vi "Proyecto Final.vi"() -> ()   [LabVIEW 2020]
panel:
  out "km":dbl
  out "ce":dbl
  out "C":dbl
  out "B":dbl
  out "A":dbl
  out "cma":dbl
  out "cpf":dbl
  out "cm":dbl
  out "F gringo":dbl
  out "ks":dbl
  in  "ks como 1":bool
  out "B":dbl
  out "A":dbl
  out "kv":dbl
  out "h gringo":dbl
  out "wt gringa":dbl
  out "v gringa":dbl
  out "dg gringo":dbl
  out "dp gringo":dbl
  out "paso gringo":dbl
  in  "ce engranajes ajusados durante el ensamble":bool
  in  "condicion":u16(ring) items=["Engranajes abiertos", "Unidades comerciales, cerradas", "Unidades de precisión, cerradas", "Unidades de precisión extrema, cerradas"]
  in  "cm op":u16(ring) items=["dientes coronados", "dientes sin coronar"]
  in  "calidad":dbl
  in  "k0":u16(ring) items=["1", "1.25", "1.5", "1.75", "2", "2.25"]
  in  "AGMA":bool
  out "poder h engrane":dbl
  out "Carga wt engrane":dbl
  out "Rall fatiga engrane":dbl
  out "Se g":dbl
  in  "kfg":dbl
  out "kbg":dbl
  out "deg":dbl
  out "tg":dbl
  out "xg":dbl
  out "Con un poder de pipñon h":dbl
  out "Carga que transmite wt piñon":dbl
  out "Rall fatiga piñon":dbl
  out "h otro salon":dbl
  out "wt salon otro":dbl
  out "potencia que puede transmitir diseñado por flexion":dbl
  out "Carga maxima transmitida wt":dbl
  out "radm":dbl
  out "kf":dbl
  out "q final":dbl
  in  "q propuesto":dbl
  out "q calculado":dbl
  in  "que q vas a utilizar":bool
  out "kt final":dbl
  in  "kt propuesto":dbl
  out "kt calculado":dbl
  in  "que kt vas a utilizar":bool
  out "r/d":dbl
  out "rf":dbl
  out "Se":dbl
  out "kb":dbl
  out "de":dbl
  out "t":dbl
  out "ec 14.3":dbl
  out "l":dbl
  out "kaa":dbl
  out "kab":dbl
  out "ka":dbl
  out "H":dbl
  out "rc":dbl
  out "r2":dbl
  out "r1":dbl
  out "Cp":dbl
  in  "Factor de diseño":dbl
  in  "acabado superficial":u16(ring) items=["", "Esmerilado", "Maquinado o laminado en frio", "Laminado en caliente", "Como sale de la forja"]
  out "Seprima":dbl
  out "YG":dbl
  in  "Dureza Brinell":dbl
  in  "Me dan dureza":bool
  in  "Sy":dbl
  in  "Sut":dbl
  in  "me dan el paso?":bool
  out "Caso":i32
  in  "Me dan esfuerzo":bool
  in  "Me dan hp?":bool
  in  "me dan ancho de cara?":bool
  out "Redondeado tabla A-17":dbl
  out "ancho de cara final":dbl
  in  "Tabla 14-8 metrica":dbl[][](array[numeric])=[[0.0, 0.0, 0.0, 0.0, 0.0, 0.0, 0.0], [0.0, 191.0, 181.0, 179.0, 174.0, 162.0, 158.0], [0.0, 181.0, 174.0, 172.0, 168.0, 158.0, 154.0], [0.0, 179.0, 172.0, 170.0, 166.0, 156.0, 152.0], [0.0, 174.0, 168.0, 166.0, 163.0, 154.0, 149.0], [0.0, 162.0, 158.0, 156.0, 154.0, 145.0, 141.0], [0.0, 158.0, 154.0, 152.0, 149.0, 141.0, 137.0]]
  in  "Tabla 14-8 inglesa":dbl[][](array[numeric])=[[0.0, 0.0, 0.0, 0.0, 0.0, 0.0, 0.0], [0.0, 2300.0, 2180.0, 2160.0, 2100.0, 1950.0, 1900.0], [0.0, 2180.0, 2090.0, 2070.0, 2020.0, 1900.0, 1850.0], [0.0, 2160.0, 2070.0, 2050.0, 2000.0, 1880.0, 1830.0], [0.0, 2100.0, 2020.0, 2000.0, 1960.0, 1850.0, 1800.0], [0.0, 1950.0, 1900.0, 1880.0, 1850.0, 1750.0, 1700.0], [0.0, 1900.0, 1850.0, 1830.0, 1800.0, 1700.0, 1650.0]]
  in  "Material de la corona":u16(ring) items=["", "Acero", "Hierro maleable", "Hierro nodular", "Hierro fundido", "Bronce al aluminio", "Bronce al estaño"]
  in  "Material del piñon":u16(ring) items=["", "Acero", "Hierro maleable", "Hierro nodular", "Hierro fundido", "Bronce al aluminio", "Bronce al estaño"]
  out "dG":dbl
  out "paso final":dbl
  out "sigma piñon final":dbl
  out "wt final":dbl
  out "kv final":dbl
  out "Velocidad final":dbl
  out "tabla metrica cuando no te dan ancho de cara 2":string[][](table)=[["0", "0", "0", "0", "0", "0"], ["0", "0", "0", "0", "0", "0"], ["0", "0", "0", "0", "0", "0"], ["0", "0", "000", "0", "0", "0"], ["0", "0", "0", "0", "0", "0"], ["0", "0", "0", "0", "0", "0"], ["0", "0", "00", "0", "0", "0"], ["0", "0", "0", "0", "0", "0"], ["0", "0", "0", "0", "0", "0"], ["0", "0", "0", "0", "0", "0"], ["0", "0", "0", "0", "0", "0"], ["0", "0", "0", "0", "0", "0"], ["0", "0", "0", "0", "0", "0"], ["0", "0", "0", "0", "0", "0"], ["0", "0", "0", "0", "0", "0"], ["0", "0", "0", "0", "0", "0"], ["0", "0", "0", "0", "0", "00"], ["0", "0", "0", "0", "0", "0"], ["0", "0", "0", "0", "0", "0"], ["0", "0", "0", "0", "0", "0"], ["0", "0", "0", "0", "0", "0"], ["0", "0", "0", "0", "0", "0"], ["0", "0", "0", "0", "0", "0"], ["0", "0", "0", "0", "0", "0"], ["0", "0", "0", "0", "0", "0"], ["0", "0", "0", "0", "0", "0"], ["0", "0", "0", "0", "0", "0"], ["0", "0", "0", "0", "0", "0"], ["0", "0", "00", "0", "0", "0"], ["0", "0", "0", "0", "0", "0"], ["0", "0", "0", "0", "0", "0"]]
  in  "Comenzar calculos":bool
  out "Indice tabla":dbl
  in  "Paso predeterminado":dbl
  out "tabla ingles cuando no te dan ancho de cara":string[][](table)=[["0", "0", "0", "0", "0", "0"], ["0", "0", "0", "0", "0", "0"], ["0", "0", "0", "0", "0", "0"], ["0", "0", "000", "0", "0", "0"], ["0", "0", "0", "0", "0", "0"], ["0", "0", "0", "0", "0", "0"], ["0", "0", "00", "0", "0", "0"], ["0", "0", "0", "0", "0", "0"], ["0", "0", "0", "0", "0", "0"], ["0", "0", "0", "0", "0", "0"], ["0", "0", "0", "0", "0", "0"], ["0", "0", "0", "0", "0", "0"], ["0", "0", "0", "0", "0", "0"], ["0", "0", "0", "0", "0", "0"], ["0", "0", "0", "0", "0", "0"], ["0", "0", "0", "0", "0", "0"], ["0", "0", "0", "0", "0", "00"], ["0", "0", "0", "0", "0", "0"], ["0", "0", "0", "0", "0", "0"], ["0", "0", "0", "0", "0", "0"], ["0", "0", "0", "0", "0", "0"], ["0", "0", "0", "0", "0", "0"], ["0", "0", "0", "0", "0", "0"], ["0", "0", "0", "0", "0", "0"], ["0", "0", "0", "0", "0", "0"], ["0", "0", "0", "0", "0", "0"], ["0", "0", "0", "0", "0", "0"], ["0", "0", "0", "0", "0", "0"], ["0", "0", "00", "0", "0", "0"], ["0", "0", "0", "0", "0", "0"], ["0", "0", "0", "0", "0", "0"]]
  out "edfuerxo on":bool
  out "Ancho de cara":dbl
  in  "Esfuerzo permisible":dbl
  in  "stop":bool
  out "Sigma piñon":dbl
  out "Wt":dbl
  out "Kv":dbl
  out "Velocidad":dbl
  out "dp":dbl
  in  "ancho de cara 2":dbl
  in  "hp":dbl
  in  "rpm":dbl
  in  "paso diametral piñon":dbl
  in  "Unidades":T1(radio)
  out "factor de forma de lewizs":string
  out "Y":dbl
  out "resultado dp":string
  out "ancho de cara":string
  in  "dientes corona":dbl
  out "dientes de la corona":string
  out "hp":string
  out "velocidad del piñon":string
  in  "angulo":dbl
  out "angulo":string
  in  "dientes piñon":sgl
  out "dientes del piñon":string
  out "Paso":string
  out "Piñon/corona":string
  # "en watts"
  # "esfuerzo de compresion"
  # "allowable bending stress"
  # "Sensibilidad a la muesca"
  # "esfuerzo admisible"
  # "cosas para sacar kt"
  # "desgaste piñon y engrane"
  # "kc=1"
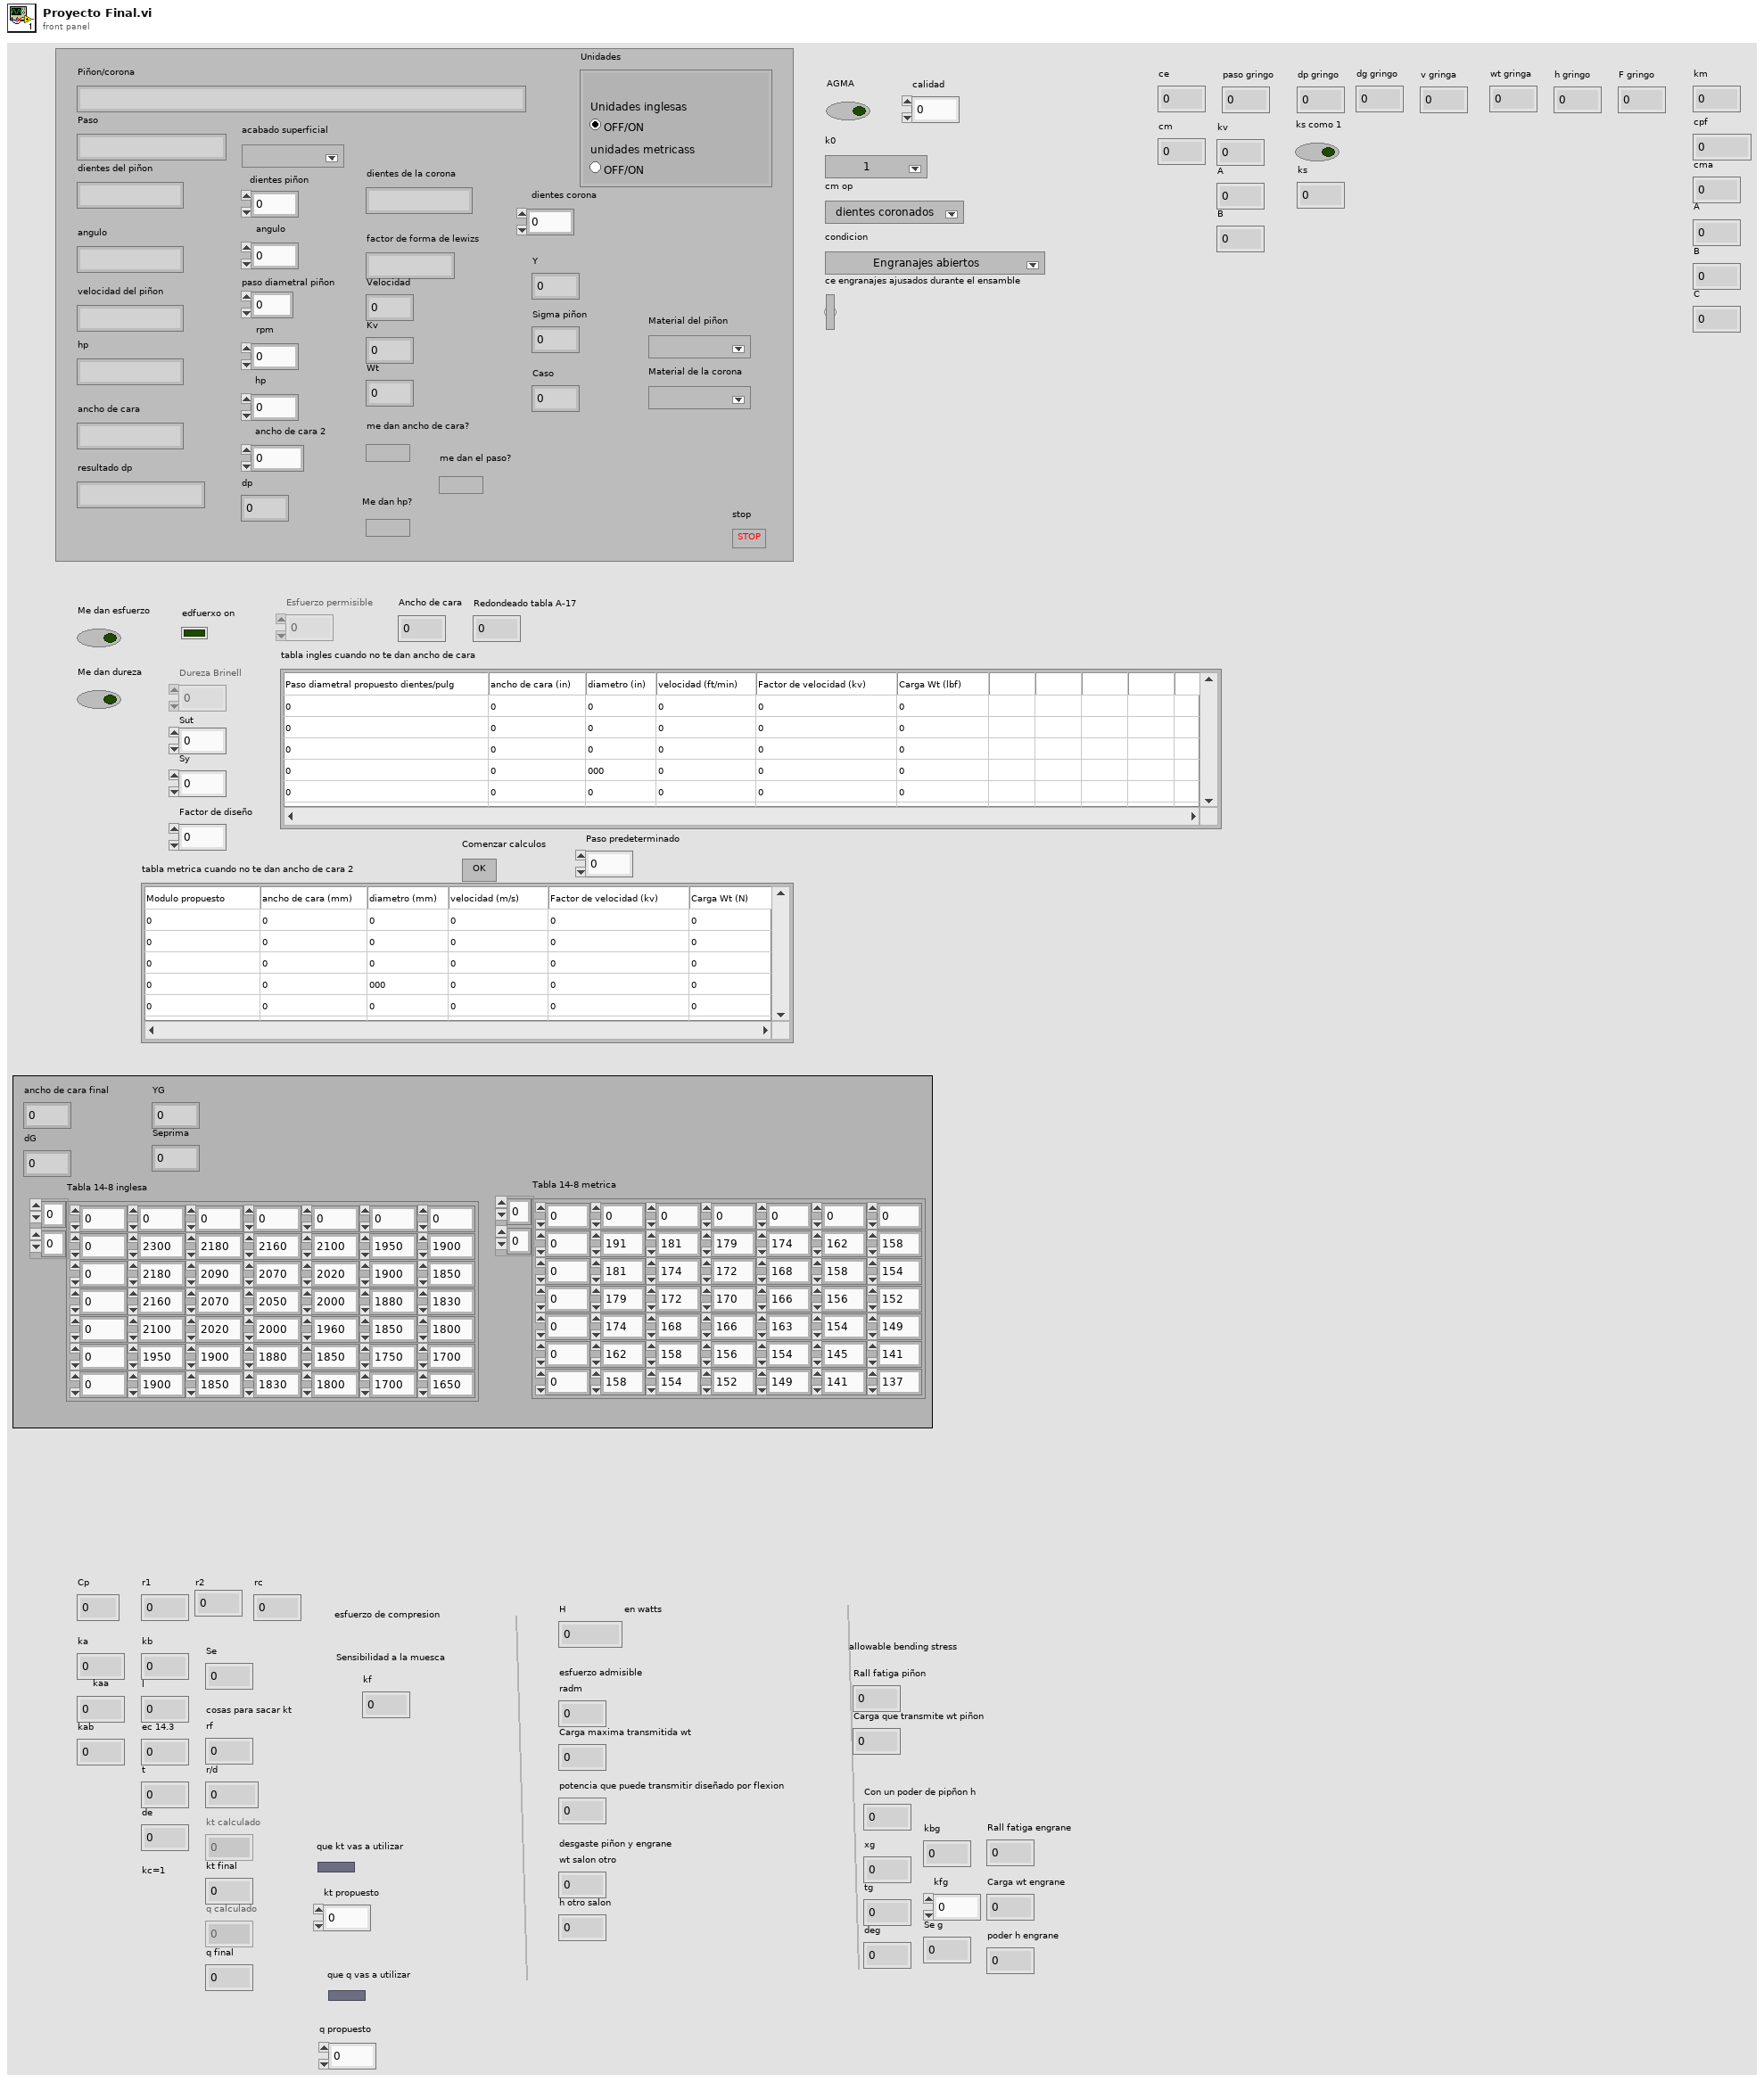
[diagram p1: front panel]
types:
  T1 = enum32{"Unidades inglesas", "unidades metricass"}
  T2 = enum8{"Enabled", "Disabled", "Disabled and Grayed Out"}
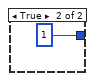
[diagram p2: hidden frame]
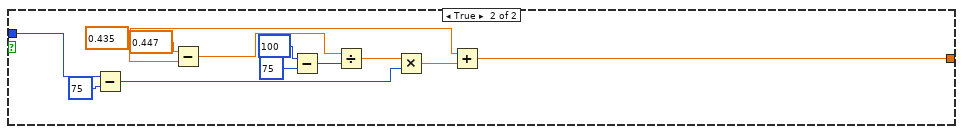
[diagram p3: hidden frame]
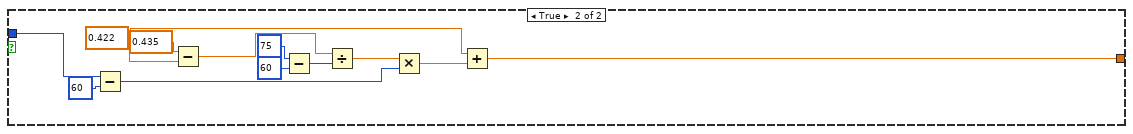
[diagram p4: hidden frame]
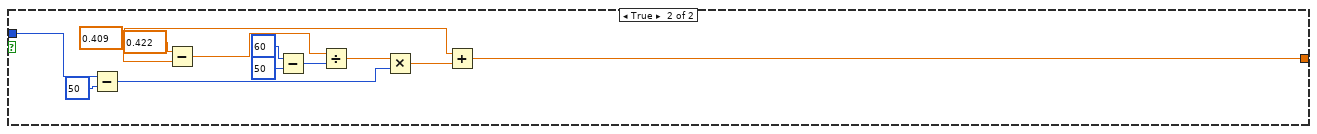
[diagram p5: hidden frame]
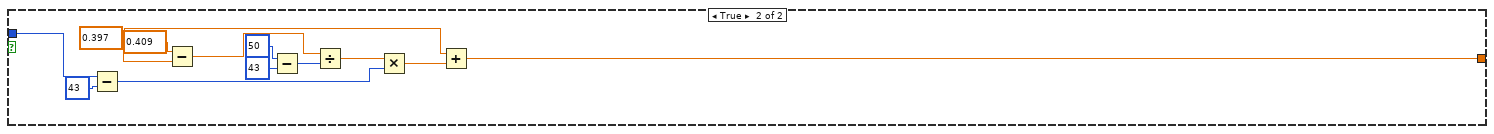
[diagram p6: hidden frame]
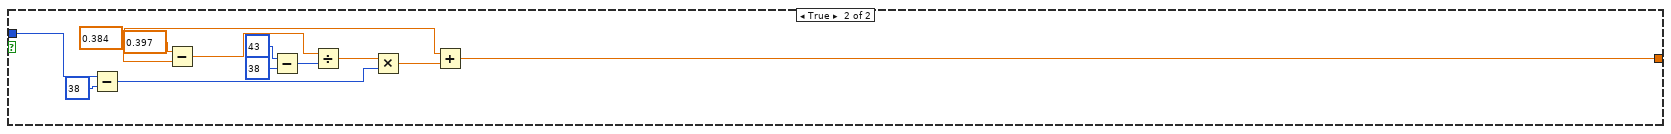
[diagram p7: hidden frame]
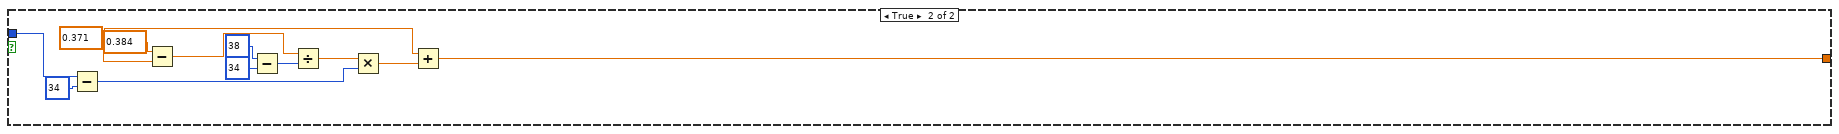
[diagram p8: hidden frame]
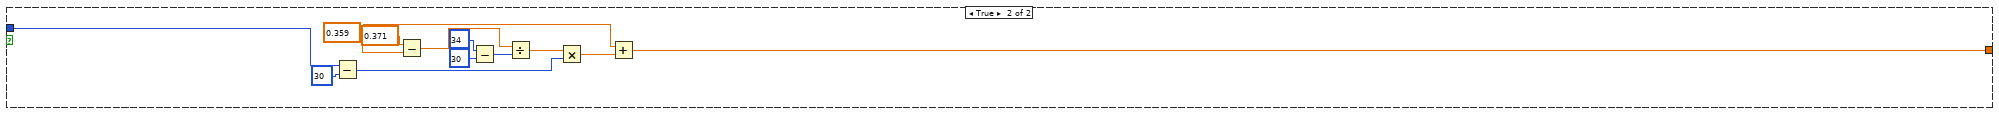
[diagram p9: hidden frame]
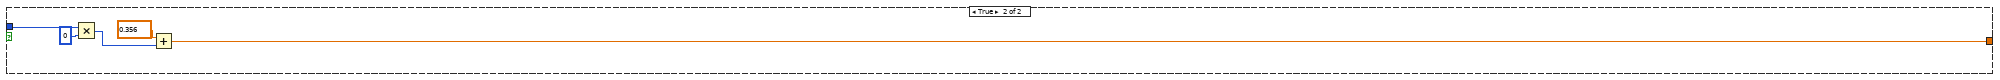
[diagram p10: hidden frame]
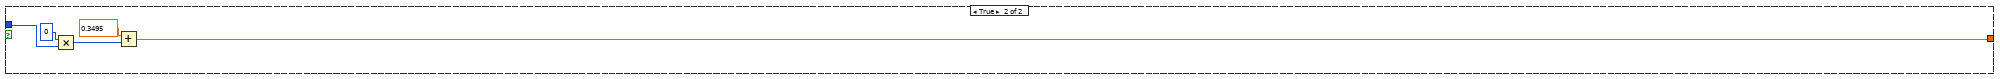
[diagram p11: hidden frame]
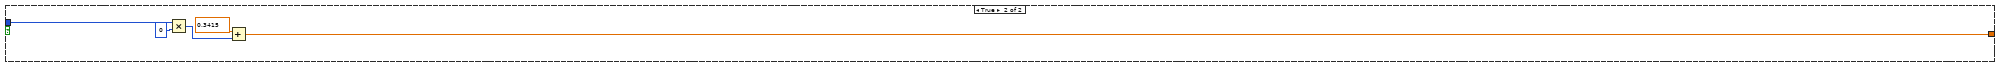
[diagram p12: hidden frame]
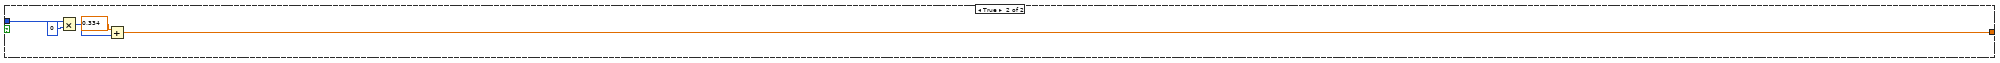
[diagram p13: hidden frame]
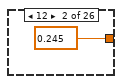
[diagram p14: hidden frame]
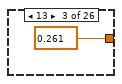
[diagram p15: hidden frame]
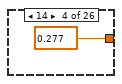
[diagram p16: hidden frame]
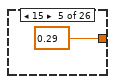
[diagram p17: hidden frame]
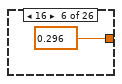
[diagram p18: hidden frame]
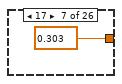
[diagram p19: hidden frame]
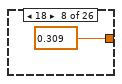
[diagram p20: hidden frame]
diagram:
  n1 = while {
    stop <- "stop" stop-if-true
    # "como lo estoy resolviendo"
    # "Caso: 0 - Me dan todos los datos\nCaso: 1 - No me dan ancho de cara\ncaso 2 - no me dan ni ancho de cara ni paso\ncaso 3 - no me dan hp"
    # "Obtengo Cp y mas cosas"
    # "Me dan todos los datos/no ocupo el sigma extra"
    # "FActor de forma de lewis final"
    # "----------------------------------------------------------------------------------------------------------------------------------------------------------------------------------------------------------------------------------------------------------------------"
    # "Seccion 14-2"
    # "---------------------------------------------------------------------------------------------------------------------------------------------------------------------------------------------------------------------"
    # "DECIDIR CUALES SON LOS DATOS BUENOS"
    # "2 Calculo factor de forma de lewis"
    n2 = local read "Wt"() -> (→"wt final":dbl)
    n3 = local read "Kv"() -> (→"kv final":dbl)
    n4 = local read "Velocidad"() -> (→"Velocidad final":dbl)
    n5 = local read "ancho de cara 2"() -> (→"ancho de cara final":dbl)
    n6 = local read "dientes corona"() -> (w44:dbl)
    n7 = property on="kv final" class="DigNum (strict)"("Visible"=FALSE) -> ()  [unwired: 2 in, 2 out]
    n8 = property on="wt final" class="DigNum (strict)"("Visible"=FALSE) -> ()  [unwired: 2 in, 2 out]
    n9 = property on="paso final" class="DigNum (strict)"("Visible"=FALSE) -> ()  [unwired: 2 in, 2 out]
    n10 = property on="sigma piñon final" class="DigNum (strict)"("Visible"=FALSE) -> ()  [unwired: 2 in, 2 out]
    n11 = property on="Velocidad final" class="DigNum (strict)"("Visible"=FALSE) -> ()  [unwired: 2 in, 2 out]
    n12 = local read "Sigma piñon"() -> (→"sigma piñon final":dbl)
    n13 = local read "paso final"() -> (w43:dbl)
    n14 = local read "Unidades"() -> (w12:T1)
    n15 = local read "angulo"() -> (w40:dbl)
    n16 = local read "dp"() -> (w41:dbl)
    n17 = local read "paso diametral piñon"() -> (→"paso final":dbl)
    n18 = case shown="\"unidades metricass\"" w12 {
      tunnel: w44 -> [w298 w302]
      tunnel: w43 -> [w299 w301]
      tunnel: [w297 w300] -> w13
      frame "Unidades inglesas", Default {
        n19 = formula code="dg=Ng/p;"("p"=w299, "Ng"=w298) -> ("dg"=w297:dbl)
      }
      frame "unidades metricass" {
        # "calcular dg"
        n20 = formula code="dg=Ng*p;"("p"=w301, "Ng"=w302) -> ("dg"=w300:dbl)
      }
    }
    "dG" <- w13
    n21 = local read "dG"() -> (w42:dbl)
    n22 = local read "Caso"() -> (w25:i32)
    n23 = case shown="\"unidades metricass\"" w12 {
      tunnel: "Material de la corona" -> [w974 w985]
      tunnel: "Material del piñon" -> [w975 w984]
      tunnel: [w973 w983] -> w45
      tunnel: w42 -> [w972 w981]
      tunnel: w41 -> [w971 w982]
      tunnel: [w970 w978] -> w46
      tunnel: [w969 w977] -> w47
      tunnel: w40 -> [w967 w980]
      frame "Unidades inglesas", Default {
        n24 = formula code="r1=dp*sin(PHI*(pip/180))/2;\nr2=dg*sin(PHI*(pip/180))/2;"("dg"=w972, "dp"=w971, "PHI"=w967, "pip"=3.141592653589793) -> ("r1"=w970:dbl, "r2"=w969:dbl)
        n25 = Index Array(array="Tabla 14-8 inglesa", index (row)=w975, index (col)=w974) -> (element=w973:dbl)
      }
      frame "unidades metricass" {
        n26 = formula code="r1=dp*sin(PHI*(pip/180))/2;\nr2=dg*sin(PHI*(pip/180))/2;"("dg"=w981, "dp"=w982, "PHI"=w980, "pip"=3.141592653589793) -> ("r1"=w978:dbl, "r2"=w977:dbl)
        n27 = Index Array(array="Tabla 14-8 metrica", index (row)=w984, index (col)=w985) -> (element=w983:dbl)
      }
    }
    "r2" <- w47
    "r1" <- w46
    "Cp" <- w45
    n28 = local read "paso diametral piñon"() -> (w21:dbl)
    n29 = local read "hp"() -> (w22:dbl)
    n30 = local read "Unidades"() -> (w1:T1)
    n31 = case shown="5" w25 {
      tunnel: w1 -> [_ w449 _ _ _ _]
      frame 0, Default {
        # "esfuerzo de compresion"
        n32 = local read "paso diametral piñon"() -> (w367:dbl)
        n33 = local read "ancho de cara 2"() -> (w369:dbl)
        n34 = local read "ancho de cara final"() -> (w362:dbl)
        n35 = local read "Unidades"() -> (w370:T1)
        n36 = local read "kv final"() -> (w359:dbl)
        n37 = local read "Y"() -> (w368:dbl)
        n38 = local read "wt final"() -> (w360:dbl)
        n39 = local read "Wt"() -> (w366:dbl)
        n40 = local read "Kv"() -> (w365:dbl)
        n41 = local read "angulo"() -> (w356:dbl)
        n42 = local read "r1"() -> (w357:dbl)
        n43 = local read "r2"() -> (w358:dbl)
        n44 = local read "Cp"() -> (w355:dbl)
        n45 = case shown="\"unidades metricass\"" w370 {
          tunnel: [w376 w380] -> w364
          tunnel: w365 -> [w375 w388]
          tunnel: w366 -> [w374 w387]
          tunnel: w367 -> [w373 w384]
          tunnel: w369 -> [w372 w385]
          tunnel: w368 -> [w371 w382]
          frame "Unidades inglesas", Default {
            # "paso"
            # "ancho de cara"
            # "sigmapiño"
            # "wt"
            # "kv"
            # "Y"
            # "Paso 6 sacar el esfuerzo de flexion"
            # "Calculo sigma flexion"
            n46 = Multiply(x=w372, y=w371) -> (x*y=w377:dbl)
            n47 = Multiply(x=w375, y=w374) -> (x*y=w379:dbl)
            n48 = Multiply(x=w379, y=w373) -> (x*y=w378:dbl)
            n49 = Divide(x=w378, y=w377) -> (x/y=w376:dbl)
          }
          frame "unidades metricass" {
            # "Y"
            # "paso diametral"
            # "F"
            # "wt"
            # "kv"
            n50 = Multiply(x=w388, y=w387) -> (x*y=w386:dbl)
            n51 = Multiply(x=w384, y=w385) -> (x*y=w383:dbl)
            n52 = Multiply(x=w383, y=w382) -> (x*y=w381:dbl)
            n53 = Divide(x=w386, y=w381) -> (x/y=w380:dbl)
          }
        }
        "Sigma piñon" <- w364
        n54 = formula code="aux2=cos(zy*pip/180);\n//rc=-cp*(((kv*wt)/(f*sin(20*(pip/180)))*(1/r1+1/r2))^(0.5);\nauxiliar1=kv*wt;\nauxiliar2=(1/r1)+(1/r2);\nauxiliar3=((auxiliar1/(aux2*f))*auxiliar2);"("cp"=w355, "kv"=w359, "wt"=w360, "f"=w362, "pip"=3.141592653589793, "r1"=w357, "r2"=w358, "zy"=w356) -> ("auxiliar3"=w353:dbl)  [unwired: 3 out]
        n55 = Negate(x=w355) -> (-x=w361:dbl)
        n56 = Square Root(x=w353) -> (sqrt(x)=w352:dbl)
        n57 = Multiply(x=w361, y=w352) -> (x*y=→"rc":dbl)
      }
      frame 5 {
        n58 = local read "dientes corona"() -> (w445:dbl)
        n59 = local read "dientes piñon"() -> (w447:sgl)
        n60 = local read "paso gringo"() -> (w444:dbl)
        n61 = local read "rpm"() -> (w442:dbl)
        n62 = Subtract(x=12, y="calidad") -> (x-y=w428:dbl)
        n63 = Divide(x=2.0, y=3.0) -> (x/y=w427:dbl)
        n64 = Multiply(x=w442, y=3.141592653589793) -> (x*y=w441:dbl)
        n65 = case shown="True" "ks como 1" {
          tunnel: [w466 1] -> w409
          frame False {
            n66 = local read "Y"() -> (w472:dbl)
            n67 = local read "F gringo"() -> (w473:dbl)
            n68 = Square Root(x=w472) -> (sqrt(x)=w474:dbl)
            n69 = local read "paso gringo"() -> (w470:dbl)
            n70 = Multiply(x=w473, y=w474) -> (x*y=w471:dbl)
            n71 = Divide(x=w471, y=w470) -> (x/y=w469:dbl)
            n72 = Power Of X(1:w469, 2:0.0535 ("y")) -> (0:w468:dbl)
            n73 = Multiply(x=1.192, y=w468) -> (x*y=w466:dbl)
          }
          frame True {
          }
        }
        "ks" <- w409
        n74 = case shown="0, Default" "cm op" {
          tunnel: [0.8 1] -> w392
          frame 0, Default {
          }
          frame 1 {
          }
        }
        "cm" <- w392
        n75 = case shown="False" "ce engranajes ajusados durante el ensamble" {
          tunnel: [1 0.8] -> w398
          frame False {
          }
          frame True {
          }
        }
        "ce" <- w398
        n76 = Power Of X(1:w428, 2:w427) -> (0:w424:dbl)
        n77 = Multiply(x=0.25, y=w424) -> (x*y=w416:dbl)
        "B" <- w416
        n78 = Divide(x=w447, y=w444) -> (x/y=w440:dbl)
        "dp gringo" <- w440
        n79 = Multiply(x=w440, y=w441) -> (x*y=w439:dbl)
        n80 = Divide(x=w439, y=12) -> (x/y=w433:dbl)
        "v gringa" <- w433
        n81 = local read "v gringa"() -> (w412:dbl)
        n82 = Divide(x=w445, y=w444) -> (x/y=→"dg gringo":dbl)
        n83 = Square Root(x=w412) -> (sqrt(x)=w413:dbl)
        n84 = local read "h gringo"() -> (w435:dbl)
        n85 = case shown="\"Unidades inglesas\", Default" w449 {
          tunnel: [w479 w486] -> w448
          tunnel: [w478 w484] -> w436
          tunnel: [w477 w480] -> w408
          frame "Unidades inglesas", Default {
            n86 = local read "paso diametral piñon"() -> (w479:dbl)
            n87 = local read "ancho de cara 2"() -> (w477:dbl)
            n88 = local read "hp"() -> (w478:dbl)
          }
          frame "unidades metricass" {
            # "conviertes todo a inglesas para no batallar"
            n89 = local read "paso diametral piñon"() -> (w488:dbl)
            n90 = local read "hp"() -> (w485:dbl)
            n91 = Multiply(x=25.4, y=w488) -> (x*y=w486:dbl)
            n92 = Multiply(x=w485, y=1.34102) -> (x*y=w484:dbl)
            n93 = local read "ancho de cara 2"() -> (w482:dbl)
            n94 = Divide(x=w482, y=25.4) -> (x/y=w480:dbl)
          }
        }
        "paso gringo" <- w448
        "h gringo" <- w436
        "F gringo" <- w408
        n95 = Subtract(x=1.0, y=w416) -> (x-y=w422:dbl)
        n96 = Multiply(x=w422, y=56) -> (x*y=w420:dbl)
        n97 = local read "A"() -> (w414:dbl)
        n98 = Add(x=w413, y=w414) -> (x+y=w411:dbl)
        n99 = Add(x=w420, y=50) -> (x+y=→"A":dbl)
        n100 = Multiply(x=33000, y=w435) -> (x*y=w434:dbl)
        n101 = Divide(x=w411, y=w414) -> (x/y=w415:dbl)
        n102 = Divide(x=w434, y=w433) -> (x/y=→"wt gringa":dbl)
        n103 = case shown="0, Default" "condicion" {
          tunnel: [0.247 0.127 0.0675 0.0036] -> w405
          tunnel: [0.0167 0.0158 0.0128 0.0102] -> w404
          tunnel: [-7.65e-05 -9.3e-05 -9.26e-05 -8.22e-05] -> w403
          frame 0, Default {
          }
          frame 1 {
          }
          frame 2 {
          }
          frame 3 {
          }
        }
        "A" <- w405
        "B" <- w404
        "C" <- w403
        n104 = local read "dp gringo"() -> (w389:dbl)
        n105 = local read "F gringo"() -> (w402:dbl)
        n106 = Power Of X(1:w415, 2:w416) -> (0:→"kv":dbl)
        n107 = formula code="if(f<=1){\ncpf=(f/(10*d))-0.025;}\nelse{\nif(f<=17){\ncpf=(f/(10*d))-0.0375+(0.0125*f);\n}else{\ncpf=(f/(10*d))-0.1109+(0.0207*f)-(0.000228*f*f);\n}\n}"("f"=w402, "d"=w389) -> ("cpf"=w396:dbl)
        "cpf" <- w396
        n108 = formula code="cma=a+(b*f)+(c*f*f);"("a"=w405, "b"=w404, "c"=w403, "f"=w402) -> ("cma"=w399:dbl)
        "cma" <- w399
        n109 = Multiply(x=w396, y=1) -> (x*y=w394:dbl)
        n110 = Multiply(x=w399, y=w398) -> (x*y=w397:dbl)
        n111 = Add(x=w397, y=w394) -> (x+y=w393:dbl)
        n112 = Multiply(x=w393, y=w392) -> (x*y=w391:dbl)
        n113 = Add(x=1.0, y=w391) -> (x+y=→"km":dbl)
      }
      frame 2 {
        # "si no me dan ancho de cara"
        n114 = case shown="True" "Comenzar calculos" {
          frame False {
          }
          frame True {
            n115 = for {
              N: 30 -> [_]
              i -> [w493]
              # "lo hace invisible"
              n116 = local read "Indice tabla"() -> (w495:dbl)
              n117 = local read "Unidades"() -> (w491:T1)
              n118 = Wait Until Next ms Multiple(millisecond multiple=u32 100) -> ()  [unwired: 1 out]
              n119 = property on="Indice tabla" class="DigNum (strict)"("Visible"=FALSE) -> ()  [unwired: 2 in, 2 out]
              n120 = case shown="\"Unidades inglesas\", Default" w491 {
                tunnel: w495 -> [w496 _]
                frame "Unidades inglesas", Default {
                  # "ancho cara"
                  # "kv"
                  # "carga"
                  # "velocidad"
                  # "paso"
                  # "sistema ingles"
                  n121 = Add(x="Paso predeterminado", y=w496) -> (x+y=w497:dbl)
                  n122 = local read "Esfuerzo permisible"() -> (w501:dbl)
                  n123 = local read "dientes piñon"() -> (w518:sgl)
                  n124 = Multiply(x=w501, y=1000) -> (x*y=w500:dbl)
                  n125 = local read "rpm"() -> (w513:dbl)
                  n126 = local read "hp"() -> (w509:dbl)
                  n127 = local read "Y"() -> (w502:dbl)
                  n128 = formula code="dp=Np/Pd;\nV=(pip*dp*n)/12;\nWt=33000*(H/V);\nkv=(V+1200)/1200;\nF=(kv*Wt*Pd)/(rb*Y);"("Pd"=w497, "Np"=w518, "pip"=3.141592653589793, "n"=w513, "H"=w509, "rb"=w500, "Y"=w502) -> ("dp"=w520:dbl, "V"=w515:dbl, "Wt"=w510:dbl, "kv"=w506:dbl, "F"=w503:dbl)
                  n129 = local read "tabla ingles cuando no te dan ancho de cara"() -> (w525:string[][])
                  n130 = Number To Fractional String(number=w497) -> (F-format string=w523:string)  [unwired: 3 in]
                  n131 = Number To Fractional String(number=w520) -> (F-format string=w519:string)  [unwired: 3 in]
                  n132 = Number To Fractional String(number=w515) -> (F-format string=w516:string)  [unwired: 3 in]
                  n133 = Number To Fractional String(number=w510) -> (F-format string=w511:string)  [unwired: 3 in]
                  n134 = Number To Fractional String(number=w506) -> (F-format string=w507:string)  [unwired: 3 in]
                  n135 = Number To Fractional String(number=w503) -> (F-format string=w504:string)  [unwired: 3 in]
                  n136 = Replace Array Subset "Replace Array Subset"(array=w525, new element #1=w523, index (row) #1=w496, index (col) #1=0 ("disabled index (col)"), new element #2=w519, index (row) #2=w496, index (col) #2=2 ("disabled index (col)"), new element #3=w516, index (row) #3=w496, index (col) #3=3, new element #4=w511, index (row) #4=w496, index (col) #4=5 ("disabled index (col)"), new element #5=w507, index (row) #5=w496, index (col) #5=4 ("disabled index (col)"), new element #6=w504, index (row) #6=w496, index (col) #6=1 ("disabled index (col)")) -> (→"tabla ingles cuando no te dan ancho de cara":string[][])
                }
                frame "unidades metricass" {
                  # "ancho cara"
                  # "kv"
                  # "carga"
                  # "velocidad"
                  # "paso"
                  # "sistema ingles"
                  n137 = local read "Esfuerzo permisible"() -> (w531:dbl)
                  n138 = local read "Paso predeterminado"() -> (w526:dbl)
                  n139 = local read "Indice tabla"() -> (w527:dbl)
                  n140 = local read "dientes piñon"() -> (w528:sgl)
                  n141 = Increment(x=w527) -> (x+1=w552:dbl)
                  n142 = Multiply(x=w531, y=1000) -> (x*y=w534:dbl)
                  n143 = feedback #1(w526) -> (w548:dbl)
                  n144 = feedback-in #1(w552) -> ()
                  n145 = local read "rpm"() -> (w529:dbl)
                  n146 = local read "hp"() -> (w530:dbl)
                  n147 = local read "Y"() -> (w532:dbl)
                  n148 = formula code="dp=Np*Pd;\nV=(pip*dp*n*0.001)/60;\nWt=(H*10000*6)/(dp*0.001*pip*n);\nkv=(V+6.1)/6.1;\nF=(kv*Wt*1000)/(rb*Y*Pd);"("Pd"=w548, "Np"=w528, "pip"=3.141592653589793, "n"=w529, "H"=w530, "rb"=w534, "Y"=w532) -> ("dp"=w550:dbl, "V"=w545:dbl, "Wt"=w541:dbl, "kv"=w538:dbl, "F"=w535:dbl)
                  n149 = local read "tabla metrica cuando no te dan ancho de cara 2"() -> (w556:string[][])
                  n150 = Number To Fractional String(number=w548) -> (F-format string=w554:string)  [unwired: 3 in]
                  n151 = Number To Fractional String(number=w550) -> (F-format string=w549:string)  [unwired: 3 in]
                  n152 = Number To Fractional String(number=w545) -> (F-format string=w546:string)  [unwired: 3 in]
                  n153 = Number To Fractional String(number=w541) -> (F-format string=w542:string)  [unwired: 3 in]
                  n154 = Number To Fractional String(number=w538) -> (F-format string=w539:string)  [unwired: 3 in]
                  n155 = Number To Fractional String(number=w535) -> (F-format string=w536:string)  [unwired: 3 in]
                  n156 = Replace Array Subset "Replace Array Subset"(array=w556, new element #1=w554, index (row) #1=w527, index (col) #1=0 ("disabled index (col)"), new element #2=w549, index (row) #2=w527, index (col) #2=2 ("disabled index (col)"), new element #3=w546, index (row) #3=w527, index (col) #3=3, new element #4=w542, index (row) #4=w527, index (col) #4=5 ("disabled index (col)"), new element #5=w539, index (row) #5=w527, index (col) #5=4 ("disabled index (col)"), new element #6=w536, index (row) #6=w527, index (col) #6=1 ("disabled index (col)")) -> (→"tabla metrica cuando no te dan ancho de cara 2":string[][])
                }
              }
              "Indice tabla" <- w493
            }
          }
        }
      }
      frame 1 {
        n157 = local read "paso diametral piñon"() -> (w562:dbl)
        n158 = local read "Esfuerzo permisible"() -> (w563:dbl)
        n159 = local read "Unidades"() -> (w557:T1)
        n160 = local read "Wt"() -> (w561:dbl)
        n161 = local read "Kv"() -> (w560:dbl)
        n162 = local read "Y"() -> (w564:dbl)
        n163 = case shown="\"Unidades inglesas\", Default" w557 {
          tunnel: w560 -> [w590 w623]
          tunnel: w561 -> [w589 w622]
          tunnel: w563 -> [w587 w620]
          tunnel: w562 -> [w588 w619]
          tunnel: w564 -> [w586 w617]
          tunnel: [w583 w615] -> w559
          frame "Unidades inglesas", Default {
            # "me dieron materiales de los engranes, ergo puedo usar r1"
            n164 = local read "Esfuerzo permisible"() -> (w584:dbl)
            n165 = local read "Cp"() -> (w585:dbl)
            n166 = local read "r2"() -> (w581:dbl)
            n167 = Greater Than 0?(x=w581) -> (x > 0?=w582:bool)
            n168 = case shown="True" w582 {
              tunnel: w590 -> [w601 w612]
              tunnel: w589 -> [w600 w611]
              tunnel: w588 -> [w598 _]
              tunnel: [w597 w602] -> w583
              tunnel: w587 -> [w596 _]
              tunnel: w586 -> [w593 _]
              tunnel: w585 -> [_ w610]
              tunnel: w584 -> [_ w608]
              frame False {
                n169 = Multiply(x=w601, y=w600) -> (x*y=w599:dbl)
                n170 = Multiply(x=1000, y=w596) -> (x*y=w592:dbl)
                n171 = Multiply(x=w599, y=w598) -> (x*y=w594:dbl)
                n172 = Multiply(x=w592, y=w593) -> (x*y=w591:dbl)
                n173 = Divide(x=w594, y=w591) -> (x/y=w597:dbl)
              }
              frame True {
                n174 = Multiply(x=w608, y=1000) -> (x*y=w606:dbl)
                n175 = Divide(x=w610, y=w606) -> (x/y=w609:dbl)
                n176 = local read "angulo"() -> (w605:dbl)
                n177 = Square(x=w609) -> (x^2=w603:dbl)
                n178 = local read "r1"() -> (w614:dbl)
                n179 = local read "r2"() -> (w613:dbl)
                n180 = formula code="invR=(1/r1)+(1/r2);\ninvA=cos(phi*pi/180);\nfrac=(kv*wt)/invA;\nDespejeC=Cuadrado*invR*frac;"("r1"=w614, "r2"=w613, "kv"=w612, "wt"=w611, "phi"=w605, "pi"=3.141592653589793, "Cuadrado"=w603) -> ("DespejeC"=w602:dbl)  [unwired: 3 out]
              }
            }
          }
          frame "unidades metricass" {
            n181 = Multiply(x=w623, y=w622) -> (x*y=w621:dbl)
            n182 = Multiply(x=w619, y=w620) -> (x*y=w618:dbl)
            n183 = Multiply(x=w618, y=w617) -> (x*y=w616:dbl)
            n184 = Divide(x=w621, y=w616) -> (x/y=w615:dbl)
          }
        }
        "Ancho de cara" <- w559
        n185 = case shown="\"unidades metricass\"" w557 {
          tunnel: w559 -> [w566 w577]
          tunnel: [w565 w575] -> w558
          frame "Unidades inglesas", Default {
            n186 = formula code="if(x<=0.01){\n    red=0.01;\n    }else{\n        if(x<=0.012){\n        red=0.012;\n        }else{\n            if(x<=0.016){\n            red=0.016;\n            }else{\n                if(x<=0.02){\n                red=0.02;\n                }else{\n                    if(x<=0.025){\n                    red=0.025;\n                    }else{\n                        if(x<=0.032){\n                        red=0.032;\n                        }else{\n                            if(x<=0.032){\n                            red=0.032;\n                            }else{\n                                if(x<=0.040){\n                                red=0.04;\n                                }else{\n                                    if(x<=0.05){\n                                    red=0.05;\n                                    }else{\n                                        if(x<=0.06){\n                                            red=0.06;\n                                        }else{\n                                            if(x<=0.08){\n                                                red=0.08;\n                                            }else{\n                                               if(x<=0.1){\n                                            red=0.1;\n                                            }else{\n                                        if(x<=0.12){\n                                        red=0.12;\n                                        }else{\n                                    if(x<=0.16){\n                                    red=0.16;\n                                    }else{\n                                if(x<=0.2){\n                                red=0.2;\n                                }else{\n                            if(x<=0.24){\n                            red=0.24;\n                            }else{\n                        if(x<=0.3){\n                        red=0.3;\n                        }else{\n                    if(x<=0.4){\n                    red=0.4;\n                    }else{\n                if(x<=0.5){\n                red=0.5;\n                }else{\n            if(x<=0.6){\n            red=0.6;\n            }else{\n        if(x<=0.8){\n        red=0.8;\n        }else{\n    if(x<=1){\n    red=1;\n    }else{\n    if(x<=1.2){\n        red=1.2;\n    }else{\n        if(x<=1.4){\n            red=1.4;\n        }else{\n            if(x<=1.6){\n                red=1.6;\n            }else{\n                if(x<=1.8){\n                    red=1.8;\n                }else{\n                    if(x<=2){\n                        red=2;\n                    }else{\n                        if(x<=2.6){\n                            red=2.6;\n                        }else{\n                            if(x<=2.8){\n                                red=2.8;\n                            }else{\n                                if(x<=3){\n                                    red=3;\n                                }else{\n                                    if(x<=3.2){\n                                    red=3.2;\n                                    }else{\n                                        if(x<=3.4){\n                                            red=3.4;\n                                        }else{\n                                            if(x<=3.6){\n                                                red=3.6;\n                                            }else{\n                                            if(x<=3.8){\n                                            red=3.8;\n                                            }else{\n                                        if(x<=4){\n                                        red=4;\n                                        }else{\n                                    if(x<=4.2){\n                                    red=4.2;\n                                    }else{\n                                if(x<=4.4){\n                                red=4.4;\n                                }else{\n                            if(x<=4.6){\n                            red=4.6;\n                            }else{\n                                red=x;\n                                        }\n                                    }\n                                }\n                            }\n                        }\n                    }\n                }\n            }\n        }\n    }                                            \n                                            }\n                                        }\n                                    }\n                                }\n                            }\n                        }\n                    }\n                }\n            }\n        }\n    } \n                                            }\n                                        }\n                                    }\n                                }\n                            }\n                        }\n                    }\n                }\n            }\n        }\n    }\n                    }}}}}}"("x"=w566) -> ("red"=w569:dbl)
            n187 = Greater?(x=w569, y=4.6) -> (0:w568:bool)
            n188 = case shown="True" w568 {
              tunnel: [w570 w572] -> w565
              tunnel: w569 -> [w570 w571]
              frame False {
              }
              frame True {
                n189 = formula code="if(x2<=4.8){\n                        red2=4.8;\n                        }else{\n                    if(x2<=5){\n                    red2=5;\n                    }else{\n                if(x2<=5.2){\n                red2=5.2;\n                }else{\n            if(x2<=5.4){\n            red2=5.4;\n            }else{\n        if(x2<=5.6){\n        red2=5.6;\n        }else{\n    if(x2<=5.8){\n    red2=5.8;\n    }else{\nif(x2<=6){\nred2=6;\n}else{\n    if(x2<=7){\n    red2=7;\n    }else{\n        if(x2<=7.5){\n        red2=7.5;\n        }else{\n            if(x2<=8.5){\n            red2=8.5;\n            }else{\n                if(x2<=9){\n                red2=9;\n                }else{\n                    if(x2<=9.5){\n                    red2=9.5;\n                    }else{\n                        if(x2<=10){\n                        red2=10;\n                        }else{\n                            if(x2<=10.5){\n                            red2=10.5;\n                            }else{\n                                if(x2<=11){\n                                red2=11;\n                                }else{\n                                    if(x2<=11.5){\n                                    red2=11.5;\n                                    }else{\n                                        if(x2<=12){\n                                        red2=12;\n                                        }else{\n                                            if(x2<=12.5){\n                                            red2=12.5;\n                                            }else{\n                                        if(x2<=13){\n                                        red2=13;\n                                        }else{\n                                    if(x2<=13.5){\n                                    red2=13.5;\n                                    }else{\n                                if(x2<=14){\n                                red2=14;\n                                }else{\n                            if(x2<=14.5){\n                            red2=14.5;\n                            }else{\n                        if(x2<=15){\n                        red2=15;\n                        }else{\n                    if(x2<=15.5){\n                    red2=15.5;\n                    }else{\n                if(x2<=16){\n                red2=16;\n                }else{\n            if(x2<=16.5){\n            red2=16.5;\n            }else{\n        if(x2<=17){\n        red2=17;\n        }else{\n    if(x2<=17.5){\n    red2=17.5;\n    }else{\nif(x2<=18){\nred2=18;\n}else{\n    if(x2<=18.5){\n    red2=18.5;   \n    }else{\n        if(x2<=19){\n        red2=19;    \n        }else{                                                \n            if(x2<=19.5){\n            red2=19.5;    \n            }else{\n            red2=20;    \n            }\n        }\n                                        }\n                                    }\n                                }\n                            }\n                        }\n                    }\n                }\n            }\n        }\n    }                                            \n                                            }\n                                        }\n                                    }\n                                }\n                            }\n                        }\n                    }\n                }\n            }\n        }\n    } \n                                            }\n                                        }\n                                    }\n                                }\n                            }\n                        }\n                    }\n                }\n            }"("x2"=w571) -> ("red2"=w572:dbl)
              }
            }
          }
          frame "unidades metricass" {
            n190 = formula code="if(x<=0.05){\n    red=0.05;\n    }else{\n        if(x<=0.06){\n        red=0.06;\n        }else{\n            if(x<=0.08){\n            red=0.08;\n            }else{\n                if(x<=0.1){\n                red=0.1;\n                }else{\n                    if(x<=0.12){\n                    red=0.12;\n                    }else{\n                        if(x<=0.16){\n                        red=0.16;\n                        }else{\n                            if(x<=0.2){\n                            red=0.2;\n                            }else{\n                                if(x<=0.25){\n                                red=0.25;\n                                }else{\n                                    if(x<=0.3){\n                                    red=0.3;\n                                    }else{\n                                        if(x<=0.4){\n                                            red=0.4;\n                                        }else{\n                                            if(x<=0.5){\n                                                red=0.5;\n                                            }else{\n                                               if(x<=0.6){\n                                            red=0.6;\n                                            }else{\n                                        if(x<=0.7){\n                                        red=0.7;\n                                        }else{\n                                    if(x<=0.8){\n                                    red=0.8;\n                                    }else{\n                                if(x<=0.9){\n                                red=0.9;\n                                }else{\n                            if(x<=1){\n                            red=1;\n                            }else{\n                        if(x<=1.1){\n                        red=1.1;\n                        }else{\n                    if(x<=1.2){\n                    red=1.2;\n                    }else{\n                if(x<=1.4){\n                red=1.4;\n                }else{\n            if(x<=1.5){\n            red=1.5;\n            }else{\n        if(x<=1.6){\n        red=1.6;\n        }else{\n    if(x<=1.8){\n    red=1.8;\n    }else{\n    if(x<=2){\n        red=2;\n    }else{\n        if(x<=2.2){\n            red=2.2;\n        }else{\n            if(x<=2.5){\n                red=2.5;\n            }else{\n                if(x<=2.8){\n                    red=2.8;\n                }else{\n                    if(x<=3){\n                        red=3;\n                    }else{\n                        if(x<=3.5){\n                            red=3.5;\n                        }else{\n                            if(x<=4){\n                                red=4;\n                            }else{\n                                if(x<=4.5){\n                                    red=4.5;\n                                }else{\n                                    if(x<=5){\n                                    red=5;\n                                    }else{\n                                        if(x<=5.5){\n                                            red=5.5;\n                                        }else{\n                                            if(x<=6){\n                                                red=6;\n                                            }else{\n                                            if(x<=6.5){\n                                            red=6.5;\n                                            }else{\n                                        if(x<=7){\n                                        red=7;\n                                        }else{\n                                    if(x<=8){\n                                    red=8;\n                                    }else{\n                                if(x<=9){\n                                red=9;\n                                }else{\n                            if(x<=10){\n                            red=10;\n                            }else{\n                                red=x;\n                                        }\n                                    }\n                                }\n                            }\n                        }\n                    }\n                }\n            }\n        }\n    }                                            \n                                            }\n                                        }\n                                    }\n                                }\n                            }\n                        }\n                    }\n                }\n            }\n        }\n    } \n                                            }\n                                        }\n                                    }\n                                }\n                            }\n                        }\n                    }\n                }\n            }\n        }\n    }\n                    }}}}}}"("x"=w577) -> ("red"=w576:dbl)
            n191 = Greater?(x=w576, y=10) -> (0:w574:bool)
            n192 = case shown="True" w574 {
              tunnel: [w578 w580] -> w575
              tunnel: w576 -> [w578 w579]
              frame False {
              }
              frame True {
                n193 = formula code="if(x2<=11){\n        red2=11;\n    }else{\n        if(x2<=12){\n        red2=12;\n        }else{\n                if(x2<=14){\n                red2=14;\n                }else{\n                    if(x2<=16){\n                    red2=16;\n                    }else{\n                        if(x2<=18){\n                        red2=18;\n                        }else{\n                            if(x2<=20){\n                            red2=20;\n                            }else{\n                                if(x2<=22){\n                                red2=22;\n                                }else{\n                                    if(x2<=25){\n                                    red2=25;\n                                    }else{\n                                        if(x2<=28){\n                                        red2=28;\n                                        }else{\n                                            if(x2<=30){\n                                            red2=30;    \n                                            }else{\n                                                if(x2<=32){\n                                                red2=32;\n                                                }else{\n                                                    if(x2<=35){\n                                                    red2=35;\n                                                    }else{\n                                                        if(x2<=40){\n                                                        red2=40;\n                                                        }else{\n                                                            if(x2<=45){\n                                                            red2=45;\n                                                            }else{\n                                                                if(x2<=50){\n                                                                red2=50;\n                                                                }else{\n                                                                    if(x2<=60){\n                                                                    red2=60;\n                                                                    }else{\n                                                                        if(x2<=80){\n                                                                        red2=80;\n                                                                        }else{\n                                                                            if(x2<=100){\n                                                                            red2=100;\n                                                                            }else{\n                                                                                if(x2<=120){\n                                                                                red2=120;\n                                                                                }else{\n                                                                                    if(x2<=140){\n                                                                                    red2=140;\n                                                                                    }else{\n                                                                                        if(x2<=160){\n                                                                                        red2=160;\n                                                                                        }else{\n                                                                                            if(x2<=180){\n                                                                                            red2=180;\n                                                                                            }else{\n                                                                                                if(x2<=200){\n                                                                                                red2=200;\n                                                                                                }else{\n                                                                                                    if(x2<=250){\n                                                                                                    red2=250;\n                                                                                                    }else{\n                                                                                                        if(x2<=300){\n                                                                                                        red2=300;\n                                                                                                        }else{\n                                                                                                            red2=x2;\n                                                                                                        }\n                                                                                                    }\n                                                                                                }\n                                                                                            }\n                                                                                        }\n                                                                                    }\n                                                                                }\n                                                                            }\n                                                                        }\n                                                                    }\n                                                                }                                            \n                                                            }\n                                                        }\n                                                    }\n                                                }\n                                            }\n                                        }\n                                    }\n                                }\n                            }\n                        }\n                    } \n                }\n            }\n        }"("x2"=w579) -> ("red2"=w580:dbl)
              }
            }
          }
        }
        "Redondeado tabla A-17" <- w558
      }
      frame 3 {
        w631 = 3.141592653589793
        # "wt"
        n194 = local read "ancho de cara 2"() -> (w625:dbl)
        n195 = local read "Unidades"() -> (w627:T1)
        n196 = local read "Esfuerzo permisible"() -> (w626:dbl)
        n197 = local read "Cp"() -> (w640:dbl)
        n198 = local read "angulo"() -> (w637:dbl)
        n199 = local read "r2"() -> (w639:dbl)
        n200 = local read "Kv"() -> (w636:dbl)
        n201 = local read "r1"() -> (w638:dbl)
        n202 = case shown="\"unidades metricass\"" w627 {
          tunnel: w625 -> [w641 w644]
          tunnel: [w641 w643] -> w624
          frame "Unidades inglesas", Default {
          }
          frame "unidades metricass" {
            n203 = Multiply(x=0.001, y=w644) -> (x*y=w643:dbl)
          }
        }
        n204 = formula code="cedos=RC/CP;\nREINV=(1/R1)+(1/R2);\npor=F*cos(PHI*pi/180);\nWet=por/(REINV*kev);"("RC"=w626, "CP"=w640, "F"=w624, "PHI"=w637, "R1"=w638, "R2"=w639, "pi"=w631, "kev"=w636) -> ("Wet"=w634:dbl, "cedos"=w635:dbl)  [unwired: 2 out]
        n205 = Square(x=w635) -> (x^2=w633:dbl)
        n206 = Multiply(x=w633, y=w634) -> (x*y=w632:dbl)
        n207 = local read "dp"() -> (w630:dbl)
        n208 = local read "rpm"() -> (w628:dbl)
        n209 = formula code="H=(wet*pi*dep*nep)/60;"("wet"=w632, "pi"=w631, "dep"=w630, "nep"=w628) -> ("H"=→"H":dbl)
      }
      frame 4 {
        # "cosas que pide el problema 14-18 --------------------------------------------------------------------------------------------------------------------------------------------------"
        # "esfuerzo permisible"
        # "ecuacion 6-32"
        # "kf = 1.66"
        # "Determinar kb"
        # "DEterminar Ka"
        n210 = local read "Factor de diseño"() -> (w653:dbl)
        n211 = local read "paso diametral piñon"() -> (w732:dbl)
        n212 = Greater Than 0?(x="Sut") -> (x > 0?=w685:bool)
        n213 = case shown="False" w685 {
          tunnel: [w751 w754] -> w684
          tunnel: "Sut" -> [_ w754]
          frame False {
            n214 = local read "Dureza Brinell"() -> (w752:dbl)
            n215 = Multiply(x=0.5, y=w752) -> (x*y=w751:dbl)
          }
          frame True {
          }
        }
        n216 = local read "Se"() -> (w678:dbl)
        n217 = local read "Seprima"() -> (w727:dbl)
        n218 = local read "kb"() -> (w726:dbl)
        n219 = local read "ka"() -> (w728:dbl)
        n220 = Multiply(x=w684, y=0.5) -> (x*y=→"Seprima":dbl)
        n221 = Multiply(x=w727, y=w728) -> (x*y=w725:dbl)
        n222 = Divide(x=w678, y=w653) -> (x/y=w677:dbl)
        "Rall fatiga piñon" <- w677
        n223 = Multiply(x=w725, y=w726) -> (x*y=w723:dbl)
        n224 = local read "paso diametral piñon"() -> (w648:dbl)
        n225 = local read "ancho de cara 2"() -> (w651:dbl)
        n226 = Multiply(x=w723, y=1.66) -> (x*y=→"Se":dbl)
        n227 = local read "Unidades"() -> (w691:T1)
        n228 = local read "Velocidad"() -> (w647:dbl)
        n229 = local read "Kv"() -> (w649:dbl)
        n230 = local read "Y"() -> (w679:dbl)
        n231 = case shown="\"Unidades inglesas\", Default" w691 {
          tunnel: [w896 w921] -> w733
          tunnel: w732 -> [w900 w927]
          tunnel: [w894 w920] -> w731
          tunnel: [w892 w918] -> w718
          tunnel: [w885 w911] -> w730
          tunnel: [w884 w913] -> w729
          frame "Unidades inglesas", Default {
            n232 = formula code="L=(1/pd)+(1.25/pd);"("pd"=w900) -> ("L"=w896:dbl)
            n233 = local read "paso diametral piñon"() -> (w898:dbl)
            n234 = local read "Y"() -> (w899:dbl)
            n235 = formula code="equis=(3*yp)/(2*pe);"("yp"=w899, "pe"=w898) -> ("equis"=w894:dbl)
            n236 = Multiply(x=4, y=w896) -> (x*y=w895:dbl)
            n237 = Multiply(x=w895, y=w894) -> (x*y=w893:dbl)
            n238 = local read "ancho de cara 2"() -> (w891:dbl)
            n239 = Square Root(x=w893) -> (sqrt(x)=w892:dbl)
            n240 = Multiply(x=w891, y=w892) -> (x*y=w890:dbl)
            n241 = Square Root(x=w890) -> (sqrt(x)=w889:dbl)
            n242 = Multiply(x=0.808, y=w889) -> (x*y=w885:dbl)
            n243 = Less Or Equal?(x=w885, y=2.0) -> (x <= y?=w887:bool)
            n244 = case shown="True" w887 {
              tunnel: w885 -> [w902 w910]
              tunnel: [w901 w906] -> w884
              frame False {
                n245 = Power Of X(1:w902, 2:-0.157 ("y")) -> (0:w904:dbl)
                n246 = Multiply(x=w904, y=0.91) -> (x*y=w901:dbl)
              }
              frame True {
                n247 = Power Of X(1:w910, 2:-0.107 ("y")) -> (0:w908:dbl)
                n248 = Multiply(x=w908, y=0.879) -> (x*y=w906:dbl)
              }
            }
          }
          frame "unidades metricass" {
            n249 = local read "paso diametral piñon"() -> (w925:dbl)
            n250 = formula code="L=(1*pd)+(1.25*pd);"("pd"=w927) -> ("L"=w921:dbl)
            n251 = local read "Y"() -> (w926:dbl)
            n252 = formula code="equis=(3*yp*pe)/2;"("yp"=w926, "pe"=w925) -> ("equis"=w920:dbl)
            n253 = Multiply(x=4, y=w921) -> (x*y=w924:dbl)
            n254 = Multiply(x=w924, y=w920) -> (x*y=w923:dbl)
            n255 = Square Root(x=w923) -> (sqrt(x)=w918:dbl)
            n256 = local read "ancho de cara 2"() -> (w919:dbl)
            n257 = Multiply(x=w919, y=w918) -> (x*y=w917:dbl)
            n258 = Square Root(x=w917) -> (sqrt(x)=w916:dbl)
            n259 = Multiply(x=0.808, y=w916) -> (x*y=w911:dbl)
            n260 = Less Or Equal?(x=w911, y=51) -> (x <= y?=w914:bool)
            n261 = case shown="False" w914 {
              tunnel: w911 -> [w929 w936]
              tunnel: [w928 w933] -> w913
              frame False {
                n262 = Power Of X(1:w929, 2:-0.157) -> (0:w930:dbl)
                n263 = Multiply(x=1.51, y=w930) -> (x*y=w928:dbl)
              }
              frame True {
                n264 = Power Of X(1:w936, 2:-0.107) -> (0:w934:dbl)
                n265 = Multiply(x=1.24, y=w934) -> (x*y=w933:dbl)
              }
            }
          }
        }
        "l" <- w733
        "ec 14.3" <- w731
        "t" <- w718
        "de" <- w730
        "kb" <- w729
        n266 = local read "paso diametral piñon"() -> (w720:dbl)
        n267 = local read "YG"() -> (w650:dbl)
        n268 = case shown="2" "acabado superficial" {
          tunnel: w691 -> [_ w941 w944 w949 w954]
          tunnel: [w938 w940 w946 w951 w956] -> w735
          tunnel: [w938 -0.265 -0.718 -0.995 -0.085] -> w738
          frame 0, Default {
            w938 = 0
          }
          frame 2 {
            n269 = case shown="\"Unidades inglesas\", Default" w941 {
              tunnel: [2.7 4.51] -> w940
              frame "Unidades inglesas", Default {
              }
              frame "unidades metricass" {
              }
            }
          }
          frame 3 {
            n270 = case shown="\"unidades metricass\"" w944 {
              tunnel: [14.4 57.7] -> w946
              frame "Unidades inglesas", Default {
              }
              frame "unidades metricass" {
              }
            }
          }
          frame 4 {
            n271 = case shown="\"unidades metricass\"" w949 {
              tunnel: [39.9 272] -> w951
              frame "Unidades inglesas", Default {
              }
              frame "unidades metricass" {
              }
            }
          }
          frame 1 {
            n272 = case shown="\"unidades metricass\"" w954 {
              tunnel: [1.34 1.58] -> w956
              frame "Unidades inglesas", Default {
              }
              frame "unidades metricass" {
              }
            }
          }
        }
        "kab" <- w738
        "kaa" <- w735
        n273 = formula code="wt=(F*y*rall)/(kv*pd);\nhp=(wt*v)/33;"("F"=w651, "y"=w679, "rall"=w677, "kv"=w649, "pd"=w648, "v"=w647) -> ("wt"=→"Carga que transmite wt piñon":dbl, "hp"=→"Con un poder de pipñon h":dbl)
        n274 = case shown="False" "que kt vas a utilizar" {
          tunnel: [T2."Disabled and Grayed Out" ("Disabled") T2."Enabled" ("Disabled")] -> w715
          tunnel: [T2."Enabled" ("Disabled") T2."Disabled and Grayed Out" ("Disabled")] -> w714
          tunnel: [w874 "kt propuesto"] -> w710
          frame False {
            n275 = local read "r/d"() -> (w878:dbl)
            n276 = Power Of X(1:w878, 2:-0.33333) -> (0:w876:dbl)
            n277 = Multiply(x=0.9072, y=w876) -> (x*y=w874:dbl)
            "kt calculado" <- w874
          }
          frame True {
          }
        }
        "kt final" <- w710
        n278 = case shown="\"unidades metricass\"" w691 {
          tunnel: 0.3 -> [w845 w849]
          tunnel: w720 -> [w844 w848]
          tunnel: [w846 w847] -> w719
          frame "Unidades inglesas", Default {
            n279 = Divide(x=w845, y=w844) -> (x/y=w846:dbl)
          }
          frame "unidades metricass" {
            n280 = Multiply(x=w849, y=w848) -> (x*y=w847:dbl)
          }
        }
        "rf" <- w719
        n281 = Power Of X(1:w684, 2:w738) -> (0:w736:dbl)
        n282 = Divide(x=w719, y=w718) -> (x/y=→"r/d":dbl)
        n283 = local read "Sut"() -> (w688:dbl)
        n284 = Multiply(x=w736, y=w735) -> (x*y=→"ka":dbl)
        n285 = Greater Than 0?(x=w688) -> (x > 0?=w689:bool)
        n286 = property on="kt calculado" class="DigNum (strict)"("DisabledEnum"=w714) -> ()  [unwired: 2 in, 2 out]
        n287 = property on="kt propuesto" class="DigNum (strict)"("DisabledEnum"=w715) -> ()  [unwired: 2 in, 2 out]
        n288 = case shown="True" w689 {
          tunnel: [w755 w760] -> w687
          tunnel: "Factor de diseño" -> [w756 w758]
          frame False {
            n289 = Divide(x="Sy", y=w756) -> (x/y=w755:dbl)
          }
          frame True {
            n290 = local read "Se"() -> (w762:dbl)
            n291 = local read "kf"() -> (w761:dbl)
            n292 = Multiply(x=w761, y=w758) -> (x*y=w759:dbl)
            n293 = Divide(x=w762, y=w759) -> (x/y=w760:dbl)
          }
        }
        "radm" <- w687
        n294 = case shown="False" "que q vas a utilizar" {
          tunnel: [T2."Disabled and Grayed Out" ("Disabled") T2."Enabled" ("Disabled")] -> w712
          tunnel: [T2."Enabled" ("Disabled") T2."Disabled and Grayed Out" ("Disabled")] -> w711
          tunnel: [w855 "q propuesto"] -> w709
          frame False {
            n295 = local read "Unidades"() -> (w854:T1)
            n296 = local read "Sut"() -> (w852:dbl)
            n297 = local read "rf"() -> (w851:dbl)
            n298 = case shown="\"unidades metricass\"" w854 {
              tunnel: [w864 w868] -> w853
              tunnel: w852 -> [w864 w870]
              tunnel: w851 -> [w863 w867]
              tunnel: [w863 w865] -> w850
              frame "Unidades inglesas", Default {
              }
              frame "unidades metricass" {
                n299 = Divide(x=w870, y=6.895) -> (x/y=w868:dbl)
                n300 = Divide(x=w867, y=25.4) -> (x/y=w865:dbl)
              }
            }
            n301 = Square Root(x=w850) -> (sqrt(x)=w857:dbl)
            n302 = Square(x=w853) -> (x^2=w860:dbl)
            n303 = Power Of X(1:w853, 2:3) -> (0:w859:dbl)
            n304 = formula code="Ra=0.246-(0.00308*sut1)+(0.0000151*sut2)-(0.0000000267*sut3);"("sut1"=w853, "sut2"=w860, "sut3"=w859) -> ("Ra"=w856:dbl)
            n305 = formula code="q=1/(1+(Ra/Rr));"("Rr"=w857, "Ra"=w856) -> ("q"=w855:dbl)
            "q calculado" <- w855
          }
          frame True {
          }
        }
        "q final" <- w709
        n306 = local read "paso diametral piñon"() -> (w674:dbl)
        n307 = formula code="kf=1+(q*(kt-1));"("kt"=w710, "q"=w709) -> ("kf"=→"kf":dbl)
        n308 = local read "YG"() -> (w675:dbl)
        n309 = local read "ancho de cara 2"() -> (w698:dbl)
        n310 = formula code="equis=(3*yg)/(2*pe);"("yg"=w675, "pe"=w674) -> ("equis"=w670:dbl)
        "xg" <- w670
        n311 = local read "paso diametral piñon"() -> (w696:dbl)
        n312 = local read "Y"() -> (w697:dbl)
        n313 = local read "l"() -> (w669:dbl)
        n314 = local read "Kv"() -> (w695:dbl)
        n315 = local read "Velocidad"() -> (w692:dbl)
        n316 = Multiply(x=4, y=w669) -> (x*y=w672:dbl)
        n317 = Multiply(x=w672, y=w670) -> (x*y=w671:dbl)
        n318 = local read "ancho de cara 2"() -> (w664:dbl)
        n319 = Square Root(x=w671) -> (sqrt(x)=w665:dbl)
        "tg" <- w665
        n320 = case shown="\"Unidades inglesas\", Default" w691 {
          tunnel: w698 -> [w818 w842]
          tunnel: w687 -> [w819 w837]
          tunnel: w697 -> [w817 w841]
          tunnel: w696 -> [w815 w839]
          tunnel: w695 -> [w816 w835]
          tunnel: [w812 w834] -> w694
          tunnel: [w813 w831] -> w693
          tunnel: w692 -> [w814 _]
          frame "Unidades inglesas", Default {
            n321 = Multiply(x=w819, y=w818) -> (x*y=w826:dbl)
            n322 = Multiply(x=w826, y=w817) -> (x*y=w824:dbl)
            n323 = Multiply(x=w816, y=w815) -> (x*y=w825:dbl)
            n324 = Divide(x=w824, y=w825) -> (x/y=w812:dbl)
            n325 = Multiply(x=1000, y=w812) -> (x*y=w823:dbl)
            n326 = Multiply(x=w823, y=w814) -> (x*y=w822:dbl)
            n327 = Divide(x=w822, y=33000) -> (x/y=w813:dbl)
          }
          frame "unidades metricass" {
            # "dp/2"
            n328 = local read "rpm"() -> (w830:dbl)
            n329 = local read "dp"() -> (w829:dbl)
            n330 = Multiply(x=w842, y=w841) -> (x*y=w840:dbl)
            n331 = Multiply(x=w840, y=w839) -> (x*y=w838:dbl)
            n332 = Divide(x=w829, y=2) -> (x/y=w827:dbl)
            n333 = Multiply(x=w838, y=w837) -> (x*y=w836:dbl)
            n334 = Divide(x=w836, y=w835) -> (x/y=w834:dbl)
            n335 = Multiply(x=w834, y=w830) -> (x*y=w833:dbl)
            n336 = Multiply(x=w833, y=w827) -> (x*y=w832:dbl)
            n337 = Divide(x=w832, y=9550000) -> (x/y=w831:dbl)
          }
        }
        "Carga maxima transmitida wt" <- w694
        "potencia que puede transmitir diseñado por flexion" <- w693
        n338 = Multiply(x=w664, y=w665) -> (x*y=w668:dbl)
        n339 = Square Root(x=w668) -> (sqrt(x)=w667:dbl)
        n340 = Multiply(x=0.808, y=w667) -> (x*y=w661:dbl)
        "deg" <- w661
        n341 = Less Or Equal?(x=w661, y=2.0) -> (x <= y?=w662:bool)
        n342 = local read "ancho de cara 2"() -> (w704:dbl)
        n343 = property on="q calculado" class="DigNum (strict)"("DisabledEnum"=w711) -> ()  [unwired: 2 in, 2 out]
        n344 = property on="q propuesto" class="DigNum (strict)"("DisabledEnum"=w712) -> ()  [unwired: 2 in, 2 out]
        n345 = case shown="True" w662 {
          tunnel: w661 -> [w742 w750]
          tunnel: [w741 w746] -> w660
          frame False {
            n346 = Power Of X(1:w742, 2:-0.157 ("y")) -> (0:w744:dbl)
            n347 = Multiply(x=w744, y=0.91) -> (x*y=w741:dbl)
          }
          frame True {
            n348 = Power Of X(1:w750, 2:-0.107 ("y")) -> (0:w748:dbl)
            n349 = Multiply(x=w748, y=0.879) -> (x*y=w746:dbl)
          }
        }
        "kbg" <- w660
        n350 = local read "angulo"() -> (w681:dbl)
        n351 = local read "r1"() -> (w702:dbl)
        n352 = local read "r2"() -> (w703:dbl)
        n353 = local read "Kv"() -> (w680:dbl)
        n354 = local read "Cp"() -> (w707:dbl)
        n355 = local read "Factor de diseño"() -> (w705:dbl)
        n356 = Multiply(x=w660, y="kfg") -> (x*y=w658:dbl)
        n357 = local read "Seprima"() -> (w655:dbl)
        n358 = local read "ka"() -> (w657:dbl)
        n359 = Multiply(x=w658, y=w657) -> (x*y=w656:dbl)
        n360 = Multiply(x=w656, y=w655) -> (x*y=w654:dbl)
        "Se g" <- w654
        n361 = Divide(x=w654, y=w653) -> (x/y=w652:dbl)
        "Rall fatiga engrane" <- w652
        n362 = formula code="wtg=(F*y*rall)/(kv*pd);\nhpg=(wtg*v)/33;"("F"=w651, "y"=w650, "rall"=w652, "kv"=w649, "pd"=w648, "v"=w647) -> ("wtg"=→"Carga wt engrane":dbl, "hpg"=→"poder h engrane":dbl)
        n363 = local read "Velocidad"() -> (w690:dbl)
        n364 = case shown="\"Unidades inglesas\", Default" w691 {
          tunnel: w707 -> [w772 w811]
          tunnel: "Dureza Brinell" -> [w774 w810]
          tunnel: w705 -> [w773 w804]
          tunnel: w704 -> [w771 w800]
          tunnel: w681 -> [w770 w799]
          tunnel: w703 -> [w768 w798]
          tunnel: w702 -> [w769 w797]
          tunnel: w680 -> [w767 w796]
          tunnel: 3.141592653589793 -> [w766 w795]
          tunnel: [w765 w791] -> w700
          tunnel: [w763 w789] -> w699
          tunnel: w690 -> [w764 _]
          frame "Unidades inglesas", Default {
            n365 = Multiply(x=0.4, y=w774) -> (x*y=w784:dbl)
            n366 = Subtract(x=w784, y=10) -> (x-y=w782:dbl)
            n367 = Multiply(x=w782, y=1000) -> (x*y=w780:dbl)
            n368 = Square Root(x=w773) -> (sqrt(x)=w779:dbl)
            n369 = Divide(x=w780, y=w779) -> (x/y=w778:dbl)
            n370 = formula code="cedos=RC/CP;\nREINV=(1/R1)+(1/R2);\npor=F*cos(PHI*pi/180);\nWet=por/(REINV*kev);"("RC"=w778, "CP"=w772, "F"=w771, "PHI"=w770, "R1"=w769, "R2"=w768, "pi"=w766, "kev"=w767) -> ("Wet"=w776:dbl, "cedos"=w777:dbl)  [unwired: 2 out]
            n371 = Square(x=w777) -> (x^2=w775:dbl)
            n372 = Multiply(x=w775, y=w776) -> (x*y=w765:dbl)
            n373 = formula code="H=(wet*V)/33000;"("wet"=w765, "V"=w764) -> ("H"=w763:dbl)
          }
          frame "unidades metricass" {
            n374 = Multiply(x=0.4, y=w810) -> (x*y=w808:dbl)
            n375 = Subtract(x=w808, y=10) -> (x-y=w806:dbl)
            n376 = Multiply(x=w806, y=6.89) -> (x*y=w803:dbl)
            n377 = Square Root(x=w804) -> (sqrt(x)=w802:dbl)
            n378 = Divide(x=w803, y=w802) -> (x/y=w801:dbl)
            n379 = formula code="cedos=RC/CP;\nREINV=(1/R1)+(1/R2);\npor=F*cos(PHI*pi/180);\nWet=por/(REINV*kev);"("RC"=w801, "CP"=w811, "F"=w800, "PHI"=w799, "R1"=w797, "R2"=w798, "pi"=w795, "kev"=w796) -> ("Wet"=w793:dbl, "cedos"=w794:dbl)  [unwired: 2 out]
            n380 = Square(x=w794) -> (x^2=w792:dbl)
            n381 = Multiply(x=w792, y=w793) -> (x*y=w791:dbl)
            n382 = local read "dp"() -> (w790:dbl)
            n383 = local read "rpm"() -> (w787:dbl)
            n384 = formula code="T=(wet*V)/2;\nH=(T*fast)/9.55;"("wet"=w791, "V"=w790, "fast"=w787) -> ("H"=w786:dbl)  [unwired: 1 out]
            n385 = Divide(x=w786, y=1000000.0) -> (x/y=w789:dbl)
          }
        }
        "wt salon otro" <- w700
        "h otro salon" <- w699
      }
    }
    n386 = local read "rpm"() -> (w20:dbl)
    n387 = case shown="\"unidades metricass\"" w1 {
      tunnel: ["paso diametral" "módulo"] -> w24
      tunnel: ["Fuerza que transmite" "Carga fija que soporta"] -> w23
      tunnel: w21 -> [w303 w344]
      tunnel: [w312 w323] -> w17
      tunnel: w20 -> [w311 w331]
      tunnel: [w306 w327] -> w18
      tunnel: [w310 w339] -> w10
      tunnel: w22 -> [w309 w337]
      tunnel: [w305 w329] -> w19
      tunnel: "dientes piñon" -> [w304 w322]
      frame "Unidades inglesas", Default {
        # "velocidad"
        # "dientes"
        # "dp"
        # "dp"
        # "wt"
        # "velocidad"
        # "kv"
        # "velocidad"
        # "rpm"
        # "paso"
        # "hp"
        # "Paso 5 calcular la carga tangente"
        # "Paso 4 factor de velocidad"
        # "Paso 3 sacar la velocidad ft/min"
        # "1 Calculo diametro de paso piñon"
        n388 = Divide(x=w304, y=w303) -> (x/y=w312:dbl)
        n389 = Multiply(x=33000, y=w309) -> (x*y=w313:dbl)
        n390 = Multiply(x=3.141592653589793, y=w312) -> (x*y=w318:dbl)
        n391 = Multiply(x=w318, y=w311) -> (x*y=w307:dbl)
        n392 = Divide(x=w307, y=12) -> (x/y=w306:dbl)
        n393 = Divide(x=w313, y=w306) -> (x/y=w305:dbl)
        n394 = Add(x=w306, y=1200) -> (x+y=w308:dbl)
        n395 = Divide(x=w308, y=1200) -> (x/y=w310:dbl)
      }
      frame "unidades metricass" {
        # "carga tangente"
        # "factor de velocidad"
        # "milimetros"
        # "velocidad"
        # "paso diametral"
        # "dp en metros"
        # "m"
        # "N"
        n396 = Multiply(x=w337, y=1000) -> (x*y=w335:dbl)
        n397 = Multiply(x=w322, y=w344) -> (x*y=w323:dbl)
        n398 = Multiply(x=w323, y=0.001) -> (x*y=w325:dbl)
        n399 = Multiply(x=60, y=w335) -> (x*y=w334:dbl)
        n400 = Multiply(x=w325, y=3.141592653589793) -> (x*y=w332:dbl)
        n401 = Multiply(x=w332, y=w331) -> (x*y=w330:dbl)
        n402 = Divide(x=w334, y=w330) -> (x/y=w329:dbl)
        n403 = Multiply(x=3.141592653589793, y=w325) -> (x*y=w343:dbl)
        n404 = Multiply(x=w343, y=w331) -> (x*y=w326:dbl)
        n405 = Divide(x=w326, y=60.0 ("rpm")) -> (x/y=w327:dbl)
        n406 = Add(x=w327, y=6.1) -> (x+y=w341:dbl)
        n407 = Divide(x=w341, y=6.1) -> (x/y=w339:dbl)
      }
    }
    "dp" <- w17
    "Velocidad" <- w18
    "Wt" <- w19
    "hp" <- w23
    "Paso" <- w24
    n408 = case shown="Default" "dientes piñon" {
      selector: "dientes piñon" -> [w993 _ _ _ _ _ _ _ _ _ _ _ _ _ _ _ _ _ _ _ _ _ _ _ _ _]
      tunnel: [w994 0.245 0.261 0.277 0.29 0.296 0.303 0.309 0.314 0.322 0.328 0.331 0.337 0.346 0.353 0.359 0.371 0.384 0.397 0.409 0.422 0.435 0.447 0.46 0.472 0.48] -> w61
      frame Default {
        # "interpolacion"
        n409 = Equal?(x=w993, y=23) -> (x = y?=w995:bool)
        n410 = case shown="False" w995 {
          tunnel: [w998 w1189] -> w994
          tunnel: w993 -> [w997 w1192]
          frame False {
            n411 = Equal?(x=w997, y=25) -> (x = y?=w999:bool)
            n412 = case shown="False" w999 {
              tunnel: [w1002 w1184] -> w998
              tunnel: w997 -> [w1001 w1187]
              frame False {
                n413 = Equal?(x=w1001, y=27) -> (x = y?=w1003:bool)
                n414 = case shown="False" w1003 {
                  tunnel: [w1007 w1179] -> w1002
                  tunnel: w1001 -> [w1005 w1182]
                  frame False {
                    n415 = Equal?(x=w1005, y=29) -> (x = y?=w1006:bool)
                    n416 = case shown="False" w1006 {
                      tunnel: [w1010 w1174] -> w1007
                      tunnel: w1005 -> [w1009 w1177]
                      frame False {
                        n417 = Less?(x=w1009, y=34) -> (x < y?=w1011:bool)
                        n418 = case shown="False" w1011 {
                          tunnel: w1009 -> [w1013 w1166]
                          tunnel: [w1014 w1162] -> w1010
                          frame False {
                            n419 = Less?(x=w1013, y=38) -> (x < y?=w1016:bool)
                            n420 = case shown="False" w1016 {
                              tunnel: [w1017 w1151] -> w1014
                              tunnel: w1013 -> [w1018 w1150]
                              frame False {
                                n421 = Less?(x=w1018, y=43) -> (x < y?=w1020:bool)
                                n422 = case shown="False" w1020 {
                                tunnel: [w1021 w1139] -> w1017
                                tunnel: w1018 -> [w1022 w1138]
                                frame False {
                                n423 = Less?(x=w1022, y=50) -> (x < y?=w1024:bool)
                                n424 = case shown="False" w1024 {
                                tunnel: [w1025 w1127] -> w1021
                                tunnel: w1022 -> [w1026 w1126]
                                frame False {
                                n425 = Less?(x=w1026, y=60) -> (x < y?=w1028:bool)
                                n426 = case shown="False" w1028 {
                                tunnel: [w1029 w1115] -> w1025
                                tunnel: w1026 -> [w1030 w1114]
                                frame False {
                                n427 = Less?(x=w1030, y=75) -> (x < y?=w1032:bool)
                                n428 = case shown="False" w1032 {
                                tunnel: [w1033 w1103] -> w1029
                                tunnel: w1030 -> [w1034 w1102]
                                frame False {
                                n429 = Less?(x=w1034, y=100) -> (x < y?=w1036:bool)
                                n430 = case shown="False" w1036 {
                                tunnel: [w1037 w1091] -> w1033
                                tunnel: w1034 -> [w1038 w1090]
                                frame False {
                                n431 = Less?(x=w1038, y=150) -> (x < y?=w1040:bool)
                                n432 = case shown="False" w1040 {
                                tunnel: [w1041 w1079] -> w1037
                                tunnel: w1038 -> [w1042 w1078]
                                frame False {
                                n433 = Less?(x=w1042, y=300) -> (x < y?=w1044:bool)
                                n434 = case shown="False" w1044 {
                                tunnel: [w1046 w1067] -> w1041
                                tunnel: w1042 -> [w1045 w1066]
                                frame False {
                                n435 = Less?(x=w1045, y=400) -> (x < y?=w1048:bool)
                                n436 = case shown="False" w1048 {
                                tunnel: [w1049 w1055] -> w1046
                                tunnel: w1045 -> [w1053 w1054]
                                frame False {
                                n437 = Multiply(x=0, y=w1053) -> (x*y=w1050:i32)
                                n438 = Add(x=w1050, y=0.485) -> (x+y=w1049:dbl)
                                }
                                frame True {
                                w1056 = 0.472
                                n439 = Subtract(x=w1054, y=300) -> (x-y=w1059:i32)
                                n440 = Subtract(x=0.48, y=w1056) -> (x-y=w1062:dbl)
                                n441 = Subtract(x=400, y=300) -> (x-y=w1061:i32)
                                n442 = Divide(x=w1062, y=w1061) -> (x/y=w1060:dbl)
                                n443 = Multiply(x=w1060, y=w1059) -> (x*y=w1057:dbl)
                                n444 = Add(x=w1056, y=w1057) -> (x+y=w1055:dbl)
                                }
                                }
                                }
                                frame True {
                                w1068 = 0.46
                                n445 = Subtract(x=w1066, y=150) -> (x-y=w1071:i32)
                                n446 = Subtract(x=0.472, y=w1068) -> (x-y=w1074:dbl)
                                n447 = Subtract(x=300, y=150) -> (x-y=w1073:i32)
                                n448 = Divide(x=w1074, y=w1073) -> (x/y=w1072:dbl)
                                n449 = Multiply(x=w1072, y=w1071) -> (x*y=w1069:dbl)
                                n450 = Add(x=w1068, y=w1069) -> (x+y=w1067:dbl)
                                }
                                }
                                }
                                frame True {
                                w1080 = 0.447
                                n451 = Subtract(x=w1078, y=100) -> (x-y=w1083:i32)
                                n452 = Subtract(x=0.46, y=w1080) -> (x-y=w1086:dbl)
                                n453 = Subtract(x=150, y=100) -> (x-y=w1085:i32)
                                n454 = Divide(x=w1086, y=w1085) -> (x/y=w1084:dbl)
                                n455 = Multiply(x=w1084, y=w1083) -> (x*y=w1081:dbl)
                                n456 = Add(x=w1080, y=w1081) -> (x+y=w1079:dbl)
                                }
                                }
                                }
                                frame True {
                                w1092 = 0.435
                                n457 = Subtract(x=w1090, y=75) -> (x-y=w1095:i32)
                                n458 = Subtract(x=0.447, y=w1092) -> (x-y=w1098:dbl)
                                n459 = Subtract(x=100, y=75) -> (x-y=w1097:i32)
                                n460 = Divide(x=w1098, y=w1097) -> (x/y=w1096:dbl)
                                n461 = Multiply(x=w1096, y=w1095) -> (x*y=w1093:dbl)
                                n462 = Add(x=w1092, y=w1093) -> (x+y=w1091:dbl)
                                }
                                }
                                }
                                frame True {
                                w1104 = 0.422
                                n463 = Subtract(x=w1102, y=60) -> (x-y=w1107:i32)
                                n464 = Subtract(x=0.435, y=w1104) -> (x-y=w1110:dbl)
                                n465 = Subtract(x=75, y=60) -> (x-y=w1109:i32)
                                n466 = Divide(x=w1110, y=w1109) -> (x/y=w1108:dbl)
                                n467 = Multiply(x=w1108, y=w1107) -> (x*y=w1105:dbl)
                                n468 = Add(x=w1104, y=w1105) -> (x+y=w1103:dbl)
                                }
                                }
                                }
                                frame True {
                                w1116 = 0.409
                                n469 = Subtract(x=w1114, y=50) -> (x-y=w1119:i32)
                                n470 = Subtract(x=0.422, y=w1116) -> (x-y=w1122:dbl)
                                n471 = Subtract(x=60, y=50) -> (x-y=w1121:i32)
                                n472 = Divide(x=w1122, y=w1121) -> (x/y=w1120:dbl)
                                n473 = Multiply(x=w1120, y=w1119) -> (x*y=w1117:dbl)
                                n474 = Add(x=w1116, y=w1117) -> (x+y=w1115:dbl)
                                }
                                }
                                }
                                frame True {
                                w1128 = 0.397
                                n475 = Subtract(x=w1126, y=43) -> (x-y=w1131:i32)
                                n476 = Subtract(x=0.409, y=w1128) -> (x-y=w1134:dbl)
                                n477 = Subtract(x=50, y=43) -> (x-y=w1133:i32)
                                n478 = Divide(x=w1134, y=w1133) -> (x/y=w1132:dbl)
                                n479 = Multiply(x=w1132, y=w1131) -> (x*y=w1129:dbl)
                                n480 = Add(x=w1128, y=w1129) -> (x+y=w1127:dbl)
                                }
                                }
                                }
                                frame True {
                                w1140 = 0.384
                                n481 = Subtract(x=w1138, y=38) -> (x-y=w1143:i32)
                                n482 = Subtract(x=0.397, y=w1140) -> (x-y=w1146:dbl)
                                n483 = Subtract(x=43, y=38) -> (x-y=w1145:i32)
                                n484 = Divide(x=w1146, y=w1145) -> (x/y=w1144:dbl)
                                n485 = Multiply(x=w1144, y=w1143) -> (x*y=w1141:dbl)
                                n486 = Add(x=w1140, y=w1141) -> (x+y=w1139:dbl)
                                }
                                }
                              }
                              frame True {
                                w1152 = 0.371
                                n487 = Subtract(x=w1150, y=34) -> (x-y=w1155:i32)
                                n488 = Subtract(x=0.384, y=w1152) -> (x-y=w1158:dbl)
                                n489 = Subtract(x=38, y=34) -> (x-y=w1157:i32)
                                n490 = Divide(x=w1158, y=w1157) -> (x/y=w1156:dbl)
                                n491 = Multiply(x=w1156, y=w1155) -> (x*y=w1153:dbl)
                                n492 = Add(x=w1152, y=w1153) -> (x+y=w1151:dbl)
                              }
                            }
                          }
                          frame True {
                            w1163 = 0.359
                            n493 = Subtract(x=w1166, y=30) -> (x-y=w1167:i32)
                            n494 = Subtract(x=0.371, y=w1163) -> (x-y=w1170:dbl)
                            n495 = Subtract(x=34, y=30) -> (x-y=w1169:i32)
                            n496 = Divide(x=w1170, y=w1169) -> (x/y=w1168:dbl)
                            n497 = Multiply(x=w1168, y=w1167) -> (x*y=w1164:dbl)
                            n498 = Add(x=w1163, y=w1164) -> (x+y=w1162:dbl)
                          }
                        }
                      }
                      frame True {
                        n499 = Multiply(x=w1177, y=0) -> (x*y=w1176:i32)
                        n500 = Add(x=0.356, y=w1176) -> (x+y=w1174:dbl)
                      }
                    }
                  }
                  frame True {
                    n501 = Multiply(x=0, y=w1182) -> (x*y=w1181:i32)
                    n502 = Add(x=0.3495, y=w1181) -> (x+y=w1179:dbl)
                  }
                }
              }
              frame True {
                n503 = Multiply(x=w1187, y=0) -> (x*y=w1186:i32)
                n504 = Add(x=0.3415, y=w1186) -> (x+y=w1184:dbl)
              }
            }
          }
          frame True {
            n505 = Multiply(x=w1192, y=0) -> (x*y=w1191:i32)
            n506 = Add(x=0.334, y=w1191) -> (x+y=w1189:dbl)
          }
        }
      }
      frame 12 {
      }
      frame 13 {
      }
      frame 14 {
      }
      frame 15 {
      }
      frame 16 {
      }
      frame 17 {
      }
      frame 18 {
      }
      frame 19 {
      }
      frame 20 {
      }
      frame 21 {
      }
      frame 22 {
      }
      frame 24 {
      }
      frame 26 {
      }
      frame 28 {
      }
      frame 30 {
      }
      frame 34 {
      }
      frame 38 {
      }
      frame 43 {
      }
      frame 50 {
      }
      frame 60 {
      }
      frame 75 {
      }
      frame 100 {
      }
      frame 150 {
      }
      frame 300 {
      }
      frame 400 {
      }
    }
    "Y" <- w61
    n507 = local read "Material del piñon"() -> (w11:u16)
    n508 = case shown="4" w11 {
      tunnel: w10 -> [w294 _]
      tunnel: [w294 w295] -> w9
      frame 0, Default {
        # "la que siempre usamos"
      }
      frame 4 {
        # "hierro fundido"
        n509 = local read "Velocidad"() -> (w296:dbl)
        n510 = formula code="vk=(3.05+Ve)/3.05;"("Ve"=w296) -> ("vk"=w295:dbl)
      }
    }
    "Kv" <- w9
    n511 = Not(x="Me dan esfuerzo") -> (.not. x?=w34:bool)
    n512 = case shown="False" "Me dan dureza" {
      tunnel: [T2."Disabled and Grayed Out" ("Disabled") T2."Enabled" ("Disabled")] -> w7
      tunnel: [0 1] -> w6
      frame False {
      }
      frame True {
      }
    }
    n513 = case shown="True" "me dan ancho de cara?" {
      tunnel: [T2."Enabled" ("Disabled") T2."Disabled and Grayed Out" ("Disabled")] -> w39
      tunnel: [1 0] -> w31
      frame False {
      }
      frame True {
      }
    }
    n514 = case shown="True" "Me dan hp?" {
      tunnel: [T2."Enabled" ("Disabled") T2."Disabled and Grayed Out" ("Disabled")] -> w36
      tunnel: [1 0] -> w30
      frame False {
      }
      frame True {
      }
    }
    n515 = case shown="False" "me dan el paso?" {
      tunnel: [T2."Enabled" ("Disabled") T2."Disabled and Grayed Out" ("Disabled")] -> w27
      tunnel: [1 0] -> w26
      frame False {
      }
      frame True {
      }
    }
    n516 = case shown="False" w34 {
      tunnel: [TRUE FALSE] -> w59
      tunnel: [T2."Enabled" ("Disabled") T2."Disabled and Grayed Out" ("Disabled")] -> w35
      tunnel: [1 0] -> w32
      frame False {
      }
      frame True {
      }
    }
    "edfuerxo on" <- w59
    n517 = case shown="False" "AGMA" {
      tunnel: [0 1] -> w2
      frame False {
      }
      frame True {
      }
    }
    n518 = property on="Esfuerzo permisible" class="DigNum (strict)"("DisabledEnum"=w35) -> ()  [unwired: 2 in, 2 out]
    n519 = property on="hp" class="DigNum (strict)"("DisabledEnum"=w36) -> ()  [unwired: 2 in, 2 out]
    n520 = property on="paso diametral piñon" class="DigNum (strict)"("DisabledEnum"=w27) -> ()  [unwired: 2 in, 2 out]
    n521 = property on="ancho de cara 2" class="DigNum (strict)"("DisabledEnum"=w39) -> ()  [unwired: 2 in, 2 out]
    n522 = property on="Dureza Brinell" class="DigNum (strict)"("DisabledEnum"=w7) -> ()  [unwired: 2 in, 2 out]
    n523 = formula code="if(AGMA==1){calculo=5;}\nelse{\nif(e==0){\n    if(b==1){calculo=4;}\n    else{calculo=0;}\n}\nelse{\n   if(ac==0){\n         if(p==1){calculo=1;} \n         else{calculo=2;}\n    }else{\n          if(hp==0){calculo=3;}\n          else{calculo=0;}\n     }\n}\n}"("e"=w32, "ac"=w31, "hp"=w30, "p"=w26, "b"=w6, "AGMA"=w2) -> ("calculo"=→"Caso":dbl)
    n524 = case shown="Default" "dientes corona" {
      selector: "dientes corona" -> [w64 _ _ _ _ _ _ _ _ _ _ _ _ _ _ _ _ _ _ _ _ _ _ _ _ _]
      tunnel: [w65 0.245 0.261 0.277 0.29 0.296 0.303 0.309 0.314 0.322 0.328 0.331 0.337 0.346 0.353 0.359 0.371 0.384 0.397 0.409 0.422 0.435 0.447 0.46 0.472 0.48] -> w4
      frame Default {
        # "interpolacion"
        n525 = Equal?(x=w64, y=23) -> (x = y?=w66:bool)
        n526 = case shown="False" w66 {
          tunnel: [w69 w260] -> w65
          tunnel: w64 -> [w68 w263]
          frame False {
            n527 = Equal?(x=w68, y=25) -> (x = y?=w70:bool)
            n528 = case shown="False" w70 {
              tunnel: [w73 w255] -> w69
              tunnel: w68 -> [w72 w258]
              frame False {
                n529 = Equal?(x=w72, y=27) -> (x = y?=w74:bool)
                n530 = case shown="False" w74 {
                  tunnel: [w78 w250] -> w73
                  tunnel: w72 -> [w76 w253]
                  frame False {
                    n531 = Equal?(x=w76, y=29) -> (x = y?=w77:bool)
                    n532 = case shown="False" w77 {
                      tunnel: [w81 w245] -> w78
                      tunnel: w76 -> [w80 w248]
                      frame False {
                        n533 = Less?(x=w80, y=34) -> (x < y?=w82:bool)
                        n534 = case shown="False" w82 {
                          tunnel: w80 -> [w84 w237]
                          tunnel: [w85 w233] -> w81
                          frame False {
                            n535 = Less?(x=w84, y=38) -> (x < y?=w87:bool)
                            n536 = case shown="False" w87 {
                              tunnel: [w88 w222] -> w85
                              tunnel: w84 -> [w89 w221]
                              frame False {
                                n537 = Less?(x=w89, y=43) -> (x < y?=w91:bool)
                                n538 = case shown="False" w91 {
                                tunnel: [w92 w210] -> w88
                                tunnel: w89 -> [w93 w209]
                                frame False {
                                n539 = Less?(x=w93, y=50) -> (x < y?=w95:bool)
                                n540 = case shown="False" w95 {
                                tunnel: [w96 w198] -> w92
                                tunnel: w93 -> [w97 w197]
                                frame False {
                                n541 = Less?(x=w97, y=60) -> (x < y?=w99:bool)
                                n542 = case shown="False" w99 {
                                tunnel: [w100 w186] -> w96
                                tunnel: w97 -> [w101 w185]
                                frame False {
                                n543 = Less?(x=w101, y=75) -> (x < y?=w103:bool)
                                n544 = case shown="False" w103 {
                                tunnel: [w104 w174] -> w100
                                tunnel: w101 -> [w105 w173]
                                frame False {
                                n545 = Less?(x=w105, y=100) -> (x < y?=w107:bool)
                                n546 = case shown="False" w107 {
                                tunnel: [w108 w162] -> w104
                                tunnel: w105 -> [w109 w161]
                                frame False {
                                n547 = Less?(x=w109, y=150) -> (x < y?=w111:bool)
                                n548 = case shown="False" w111 {
                                tunnel: [w112 w150] -> w108
                                tunnel: w109 -> [w113 w149]
                                frame False {
                                n549 = Less?(x=w113, y=300) -> (x < y?=w115:bool)
                                n550 = case shown="False" w115 {
                                tunnel: [w117 w138] -> w112
                                tunnel: w113 -> [w116 w137]
                                frame False {
                                n551 = Less?(x=w116, y=400) -> (x < y?=w119:bool)
                                n552 = case shown="False" w119 {
                                tunnel: [w120 w126] -> w117
                                tunnel: w116 -> [w124 w125]
                                frame False {
                                n553 = Multiply(x=0, y=w124) -> (x*y=w121:i32)
                                n554 = Add(x=w121, y=0.485) -> (x+y=w120:dbl)
                                }
                                frame True {
                                w127 = 0.472
                                n555 = Subtract(x=w125, y=300) -> (x-y=w130:i32)
                                n556 = Subtract(x=0.48, y=w127) -> (x-y=w133:dbl)
                                n557 = Subtract(x=400, y=300) -> (x-y=w132:i32)
                                n558 = Divide(x=w133, y=w132) -> (x/y=w131:dbl)
                                n559 = Multiply(x=w131, y=w130) -> (x*y=w128:dbl)
                                n560 = Add(x=w127, y=w128) -> (x+y=w126:dbl)
                                }
                                }
                                }
                                frame True {
                                w139 = 0.46
                                n561 = Subtract(x=w137, y=150) -> (x-y=w142:i32)
                                n562 = Subtract(x=0.472, y=w139) -> (x-y=w145:dbl)
                                n563 = Subtract(x=300, y=150) -> (x-y=w144:i32)
                                n564 = Divide(x=w145, y=w144) -> (x/y=w143:dbl)
                                n565 = Multiply(x=w143, y=w142) -> (x*y=w140:dbl)
                                n566 = Add(x=w139, y=w140) -> (x+y=w138:dbl)
                                }
                                }
                                }
                                frame True {
                                w151 = 0.447
                                n567 = Subtract(x=w149, y=100) -> (x-y=w154:i32)
                                n568 = Subtract(x=0.46, y=w151) -> (x-y=w157:dbl)
                                n569 = Subtract(x=150, y=100) -> (x-y=w156:i32)
                                n570 = Divide(x=w157, y=w156) -> (x/y=w155:dbl)
                                n571 = Multiply(x=w155, y=w154) -> (x*y=w152:dbl)
                                n572 = Add(x=w151, y=w152) -> (x+y=w150:dbl)
                                }
                                }
                                }
                                frame True {
                                w163 = 0.435
                                n573 = Subtract(x=w161, y=75) -> (x-y=w166:i32)
                                n574 = Subtract(x=0.447, y=w163) -> (x-y=w169:dbl)
                                n575 = Subtract(x=100, y=75) -> (x-y=w168:i32)
                                n576 = Divide(x=w169, y=w168) -> (x/y=w167:dbl)
                                n577 = Multiply(x=w167, y=w166) -> (x*y=w164:dbl)
                                n578 = Add(x=w163, y=w164) -> (x+y=w162:dbl)
                                }
                                }
                                }
                                frame True {
                                w175 = 0.422
                                n579 = Subtract(x=w173, y=60) -> (x-y=w178:i32)
                                n580 = Subtract(x=0.435, y=w175) -> (x-y=w181:dbl)
                                n581 = Subtract(x=75, y=60) -> (x-y=w180:i32)
                                n582 = Divide(x=w181, y=w180) -> (x/y=w179:dbl)
                                n583 = Multiply(x=w179, y=w178) -> (x*y=w176:dbl)
                                n584 = Add(x=w175, y=w176) -> (x+y=w174:dbl)
                                }
                                }
                                }
                                frame True {
                                w187 = 0.409
                                n585 = Subtract(x=w185, y=50) -> (x-y=w190:i32)
                                n586 = Subtract(x=0.422, y=w187) -> (x-y=w193:dbl)
                                n587 = Subtract(x=60, y=50) -> (x-y=w192:i32)
                                n588 = Divide(x=w193, y=w192) -> (x/y=w191:dbl)
                                n589 = Multiply(x=w191, y=w190) -> (x*y=w188:dbl)
                                n590 = Add(x=w187, y=w188) -> (x+y=w186:dbl)
                                }
                                }
                                }
                                frame True {
                                w199 = 0.397
                                n591 = Subtract(x=w197, y=43) -> (x-y=w202:i32)
                                n592 = Subtract(x=0.409, y=w199) -> (x-y=w205:dbl)
                                n593 = Subtract(x=50, y=43) -> (x-y=w204:i32)
                                n594 = Divide(x=w205, y=w204) -> (x/y=w203:dbl)
                                n595 = Multiply(x=w203, y=w202) -> (x*y=w200:dbl)
                                n596 = Add(x=w199, y=w200) -> (x+y=w198:dbl)
                                }
                                }
                                }
                                frame True {
                                w211 = 0.384
                                n597 = Subtract(x=w209, y=38) -> (x-y=w214:i32)
                                n598 = Subtract(x=0.397, y=w211) -> (x-y=w217:dbl)
                                n599 = Subtract(x=43, y=38) -> (x-y=w216:i32)
                                n600 = Divide(x=w217, y=w216) -> (x/y=w215:dbl)
                                n601 = Multiply(x=w215, y=w214) -> (x*y=w212:dbl)
                                n602 = Add(x=w211, y=w212) -> (x+y=w210:dbl)
                                }
                                }
                              }
                              frame True {
                                w223 = 0.371
                                n603 = Subtract(x=w221, y=34) -> (x-y=w226:i32)
                                n604 = Subtract(x=0.384, y=w223) -> (x-y=w229:dbl)
                                n605 = Subtract(x=38, y=34) -> (x-y=w228:i32)
                                n606 = Divide(x=w229, y=w228) -> (x/y=w227:dbl)
                                n607 = Multiply(x=w227, y=w226) -> (x*y=w224:dbl)
                                n608 = Add(x=w223, y=w224) -> (x+y=w222:dbl)
                              }
                            }
                          }
                          frame True {
                            w234 = 0.359
                            n609 = Subtract(x=w237, y=30) -> (x-y=w238:i32)
                            n610 = Subtract(x=0.371, y=w234) -> (x-y=w241:dbl)
                            n611 = Subtract(x=34, y=30) -> (x-y=w240:i32)
                            n612 = Divide(x=w241, y=w240) -> (x/y=w239:dbl)
                            n613 = Multiply(x=w239, y=w238) -> (x*y=w235:dbl)
                            n614 = Add(x=w234, y=w235) -> (x+y=w233:dbl)
                          }
                        }
                      }
                      frame True {
                        n615 = Multiply(x=w248, y=0) -> (x*y=w247:i32)
                        n616 = Add(x=0.356, y=w247) -> (x+y=w245:dbl)
                      }
                    }
                  }
                  frame True {
                    n617 = Multiply(x=0, y=w253) -> (x*y=w252:i32)
                    n618 = Add(x=0.3495, y=w252) -> (x+y=w250:dbl)
                  }
                }
              }
              frame True {
                n619 = Multiply(x=w258, y=0) -> (x*y=w257:i32)
                n620 = Add(x=0.3415, y=w257) -> (x+y=w255:dbl)
              }
            }
          }
          frame True {
            n621 = Multiply(x=w263, y=0) -> (x*y=w262:i32)
            n622 = Add(x=0.334, y=w262) -> (x+y=w260:dbl)
          }
        }
      }
      frame 12 {
      }
      frame 13 {
      }
      frame 14 {
      }
      frame 15 {
      }
      frame 16 {
      }
      frame 17 {
      }
      frame 18 {
      }
      frame 19 {
      }
      frame 20 {
      }
      frame 21 {
      }
      frame 22 {
      }
      frame 24 {
      }
      frame 26 {
      }
      frame 28 {
      }
      frame 30 {
      }
      frame 34 {
      }
      frame 38 {
      }
      frame 43 {
      }
      frame 50 {
      }
      frame 60 {
      }
      frame 75 {
      }
      frame 100 {
      }
      frame 150 {
      }
      frame 300 {
      }
      frame 400 {
      }
    }
    "YG" <- w4
  }
